vi "Orca Flash Capture Manager.vi"(7 "Calling VI Ref":refnum<vi>) -> ()   [LabVIEW 2016]
uses:
  Orca Flash Capture Manager Controls/Orca Flash Capture Switch Line Scan Modes.ctl
  Orca Flash Capture Manager Controls/Orca Flash Capture Line Scan Settings.ctl
  Orca Flash Capture Manager Controls/Orca Flash Switch Cycles Steps.ctl
  Orca Flash Capture Manager Controls/Orca Flash Channel Element.ctl
  <vilib>/Utility/miscctls.llb/LVPointTypeDef.ctl
  Orca Flash Capture Manager Controls/Orca Flash Capture Notifier Type.ctl
  Orca Flash Capture Manager Controls/Orca Flash Capture Actions.ctl
  <vilib>/vision/Image Controls.llb/IMAQ Image.ctl
  Orca Flash Capture Manager Controls/Orca Flash Capture Line Scan Filter Settings.ctl
  Device Library/Cameras/Hamamatsu/Orca Flash/Orca Flash Controls/Orca Flash SubRegion Type.ctl
  Hardware Configuration/Hardware Configuration Controls/Device Type.ctl
  Hardware Configuration/Hardware Configuration Controls/Device Function.ctl
  Device Library/Cameras/Hamamatsu/Orca Flash/Orca Flash Controls/Orca Flash Actions.ctl
  Device Library/Cameras/Hamamatsu/Orca Flash/Orca Flash Controls/Orca Flash Parameters.ctl
  Device Library/Cameras/Hamamatsu/Orca Flash/Orca Flash Controls/Orca Flash Parameter List.ctl
  Device Library/Cameras/Hamamatsu/Orca Flash/Orca Flash Controls/Orca Flash ROI.ctl
  Orca Flash Capture Manager Controls/Orca Flash Capture Cycle Step Count.ctl
  Device Manager/Common Device Queue/Common Device Controls/Common Device Actions.ctl
  Device Library/SMTP Email Alerts/SMTP Email Alerts Type Defs/SMTP Email Alerts Actions.ctl
  Device Library/DAQmx/AO Single Channel Triggered Ramp/AO SCTR Type Defs/AO SCTR Actions.ctl
  Wide Field Drift Correction/WFDC Controls/WFDC External Sync.ctl
  Wide Field Drift Correction/WFDC Controls/WFDC Cycle Pause.ctl
  Wide Field Drift Correction/WFDC Controls/WFDC Status.ctl
  Device Library/Stages/Stages Controls/Stage Actions.ctl
  Device Library/AOTF and AOM/AOTF Controls/AOTF Actions.ctl
  Device Library/Cameras/Camera Controls/Camera IMAQ Key Info.ctl
  <vilib>/Utility/file.llb/Read Delimited Spreadsheet (DBL).vi
  shell32.dll
panel:
  in  "Main Tab":T1(tab)
  in  "Scan Mode":T2=enum."Cycles Then Steps"
  out "Frame":u32(slide) scale=0.0..3.0
  out "Cycle":sgl(slide) scale=0.0..1.0
  in  "Base Save Path":path
  in  "Capture":bool
  in  "Live Preview":bool
  out "Z Step":sgl(slide) scale=0.0..1.0
  in  "File Name":string="Test Image"
  in  "Preview Exposure Time (s)":dbl=0.1 caption="Frame Rate (Hz)"
  in  "Capture Exposure Time (s)":dbl=0.1 caption="Frame Rate (Hz)"
  in  "No. of Frames":u32=1 min=1
  in  "No. of Cycles":u16=1 min=1
  in  "No. of Z Steps":u16=1 min=1
  in  "Z Step Size (µm)":dbl min=-10.0 max=10.0
  out "Current Cycle":u16
  out "Current Step":u16
  out "Current Frame":u32
  in  "Auto Update Subfolder":bool=TRUE
  in  "Subfolder Name":string="Area"
  in  "Channel Array":T3[](array[typedef])
  in  "Channels On/Off":bool
  in  "Current Filter":i32(ring) items=["Quad Band", "Cy3 / Cy5"]
  in  "Save As Preset":bool
  in  "Line Scan Active":bool
  in  "Number of Lines":u32=8 min=1 max=200 step=1
  in  "Line Scan Mode":T4
  in  "Line Scanning Presets":u16(ring) items=["04 FPS", "08 FPS Clean", "08 FPS", "40 FPS"]
  in  "Line Scan Settings":T5
  in  "Collect Metadata":bool
  in  "Edit Metadata":bool
  in  "Camera Settings":bool
  in  "Email Alerts":bool
  in  "Email Address":string
  in  "Auto Laser Off Time (min)":u16=30
  in  "Quit":bool
  # "Live Preview"
  # "Capture"
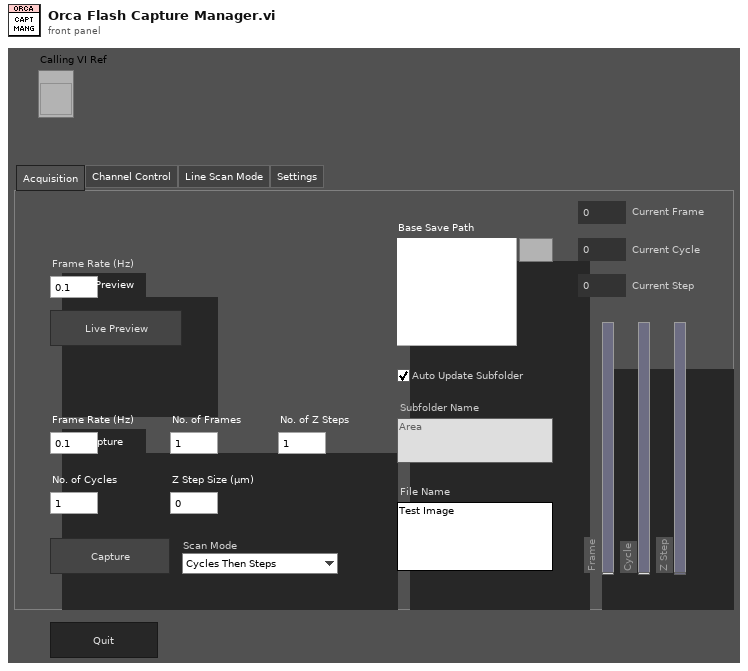
[diagram p1: front panel]
types:
  T1 = enum32{"Acquisition", "Channel Control", "Line Scan Mode", "Settings"}
  T2 = typedef "Orca Flash Switch Cycles Steps.ctl" = enum16{"Steps Then Cycles", "Cycles Then Steps"}
  T3 = typedef "Orca Flash Channel Element.ctl" = cluster{"On/Off":bool, "Name":string}
  T4 = typedef "Orca Flash Capture Switch Line Scan Modes.ctl" = enum32{"Automatic", "Use Presets", "Manual"}
  T5 = typedef "Orca Flash Capture Line Scan Settings.ctl" = cluster{"Interline Interval":dbl, "Offset (V)":dbl, "Amplitude (V)":dbl, "Samples Per Channel":dbl, "Delay (ms)":dbl}
  T6 = typedef "Orca Flash SubRegion Type.ctl" = cluster{"Name":string, "H Offset":i32, "V Offset":i32, "H Width":i32, "V Width":i32, "Active?":bool}
  T7 = typedef "IMAQ Image.ctl" = refnum<image>
  T8 = cluster{"Image Ref":T7, "Cycle Number":u16, "Camera Running?":bool, "Capture?":bool}
  T9 = typedef "Orca Flash Capture Line Scan Filter Settings.ctl" = cluster{"Filter Name":string, "Offset (V)":dbl}[]
  T10 = enum8{"Enabled", "Disabled", "Disabled and Grayed Out"}
  T11 = typedef "Orca Flash Capture Notifier Type.ctl" = cluster{"Actions":T12, "Running?":bool, "Preview Exposure (s)":dbl, "Capture Exposure (s)":dbl, "Cycles":u16, "Frames":u32, "No. of Z Steps":u16, "Z Step Size (µm)":dbl, "Base Path":path, "Init Z Position (µm)":dbl, "Save Path":path, "Line Scan?":bool, "Line Scan Mode":T4, "Collect Metadata?":bool}
  T12 = typedef "Orca Flash Capture Actions.ctl" = enum16{"Idle", "Live Preview", "Capture", "Laser On", "Laser Off", "Open Shutters", "Close Shutters", "Set Exposure Time", "Start Acquisition", "Update SubFolder", "Write Metadata", "Setup", "Camera", "Switch", "Step", "Cycle", "External Cycle Sync", "Abort", "Quit"}
  T13 = enum16{"Always On", "Always Off", "Off While Running"}
  T14 = typedef "LVPointTypeDef.ctl" = cluster{"Horizontal":i16, "Vertical":i16}
  T15 = typedef "Image Type" = u32
  T16 = typedef "Device Function.ctl" = enum16{"Primary", "Secondary", "Overview", "Wide Field Drift Correction", "642 nm Excitation", "560 nm Excitation", "546 nm Excitation", "488 nm Excitation", "405 nm Excitation", "Objective Drift Correction", "4Pi Objective Lock", "Objective XY", "Objective Z", "Sample XY", "Sample Coarse Z", "Sample Z", "4Pi Lower", "4Pi Upper", "Adj Cavity", "Line Scanning", "Alert"}
  T17 = typedef "Device Type.ctl" = enum16{"AOTF", "Camera", "Deformable Mirror", "Laser", "Shutter", "Stage", "Waveform", "Email"}
  T18 = typedef "Orca Flash ROI.ctl" = cluster{"H Offset":i32, "V Offset":i32, "H Width":i32, "V Width":i32}
  T19 = typedef "Orca Flash Parameters.ctl" = cluster{"Value":dbl, "Parameter":T20}
  T20 = typedef "Orca Flash Parameter List.ctl" = u32
  T21 = typedef "Orca Flash Actions.ctl" = enum16{"IDLE", "PREVIEW", "RECORD", "Record Settings", "SETPARAM", "GETPARAM", "SETROI", "GETROI", "PROGRESSIVE MODE", "AREA MODE", "STATUS", "QUIT"}
  T22 = typedef "Orca Flash Capture Cycle Step Count.ctl" = cluster{"Scan Mode":T2, "Current Step":u16, "Current Cycle":u16, "Num of Steps":u16, "Num of Cycles":u16}
  T23 = typedef "WFDC Status.ctl" = enum16{"Idle", "Busy", "DC Active", "Error"}
  T24 = typedef "WFDC External Sync.ctl" = cluster{"Cycle Sync":T25, "Z Offset":dbl, "WFDC Status":T23}
  T25 = typedef "WFDC Cycle Pause.ctl" = enum16{"Pause Requested", "Paused", "Resume Requested", "Resumed"}
  T26 = typedef "SMTP Email Alerts Actions.ctl" = enum16{"Set Recipient", "Send Message", "Quit"}
  T27 = typedef "Stage Actions.ctl" = enum16{"Get Position", "MVR", "MOVE", "HALT", "ONTARGET", "ERROR", "REFERENCE", "INIT", "VELOCITY", "STATUS", "EXIT", "HOME", "ZEROPOS", "NANOPOS", "ANALOG", "QUIT"}
  T28 = typedef "AOTF Actions.ctl" = enum16{"Error Check", "Blank", "Line On/Off", "Set Power", "Status", "Quit"}
  T29 = typedef "AO SCTR Actions.ctl" = enum16{"Stop at Offset", "Update and Run", "Quit"}
  T30 = typedef "Camera IMAQ Key Info.ctl" = cluster{"Frame":u32, "Sensor Height":i32, "Sensor Width":i32, "ROI Height":i32, "ROI Width":i32, "ROI Enable?":bool, "Bit per Pixel":u8}
  T31 = typedef "Common Device Actions.ctl" = enum16{"Specific Action", "Open Front Panel", "Close Front Panel", "Quit", "Quit All"}
  T32 = typedef "LVRectTypeDef.ctl" = cluster{"Left":i16, "Top":i16, "Right":i16, "Bottom":i16}
  T33 = typedef "LVBoundsTypeDef.ctl" = cluster{"Width":u32, "Height":u32}
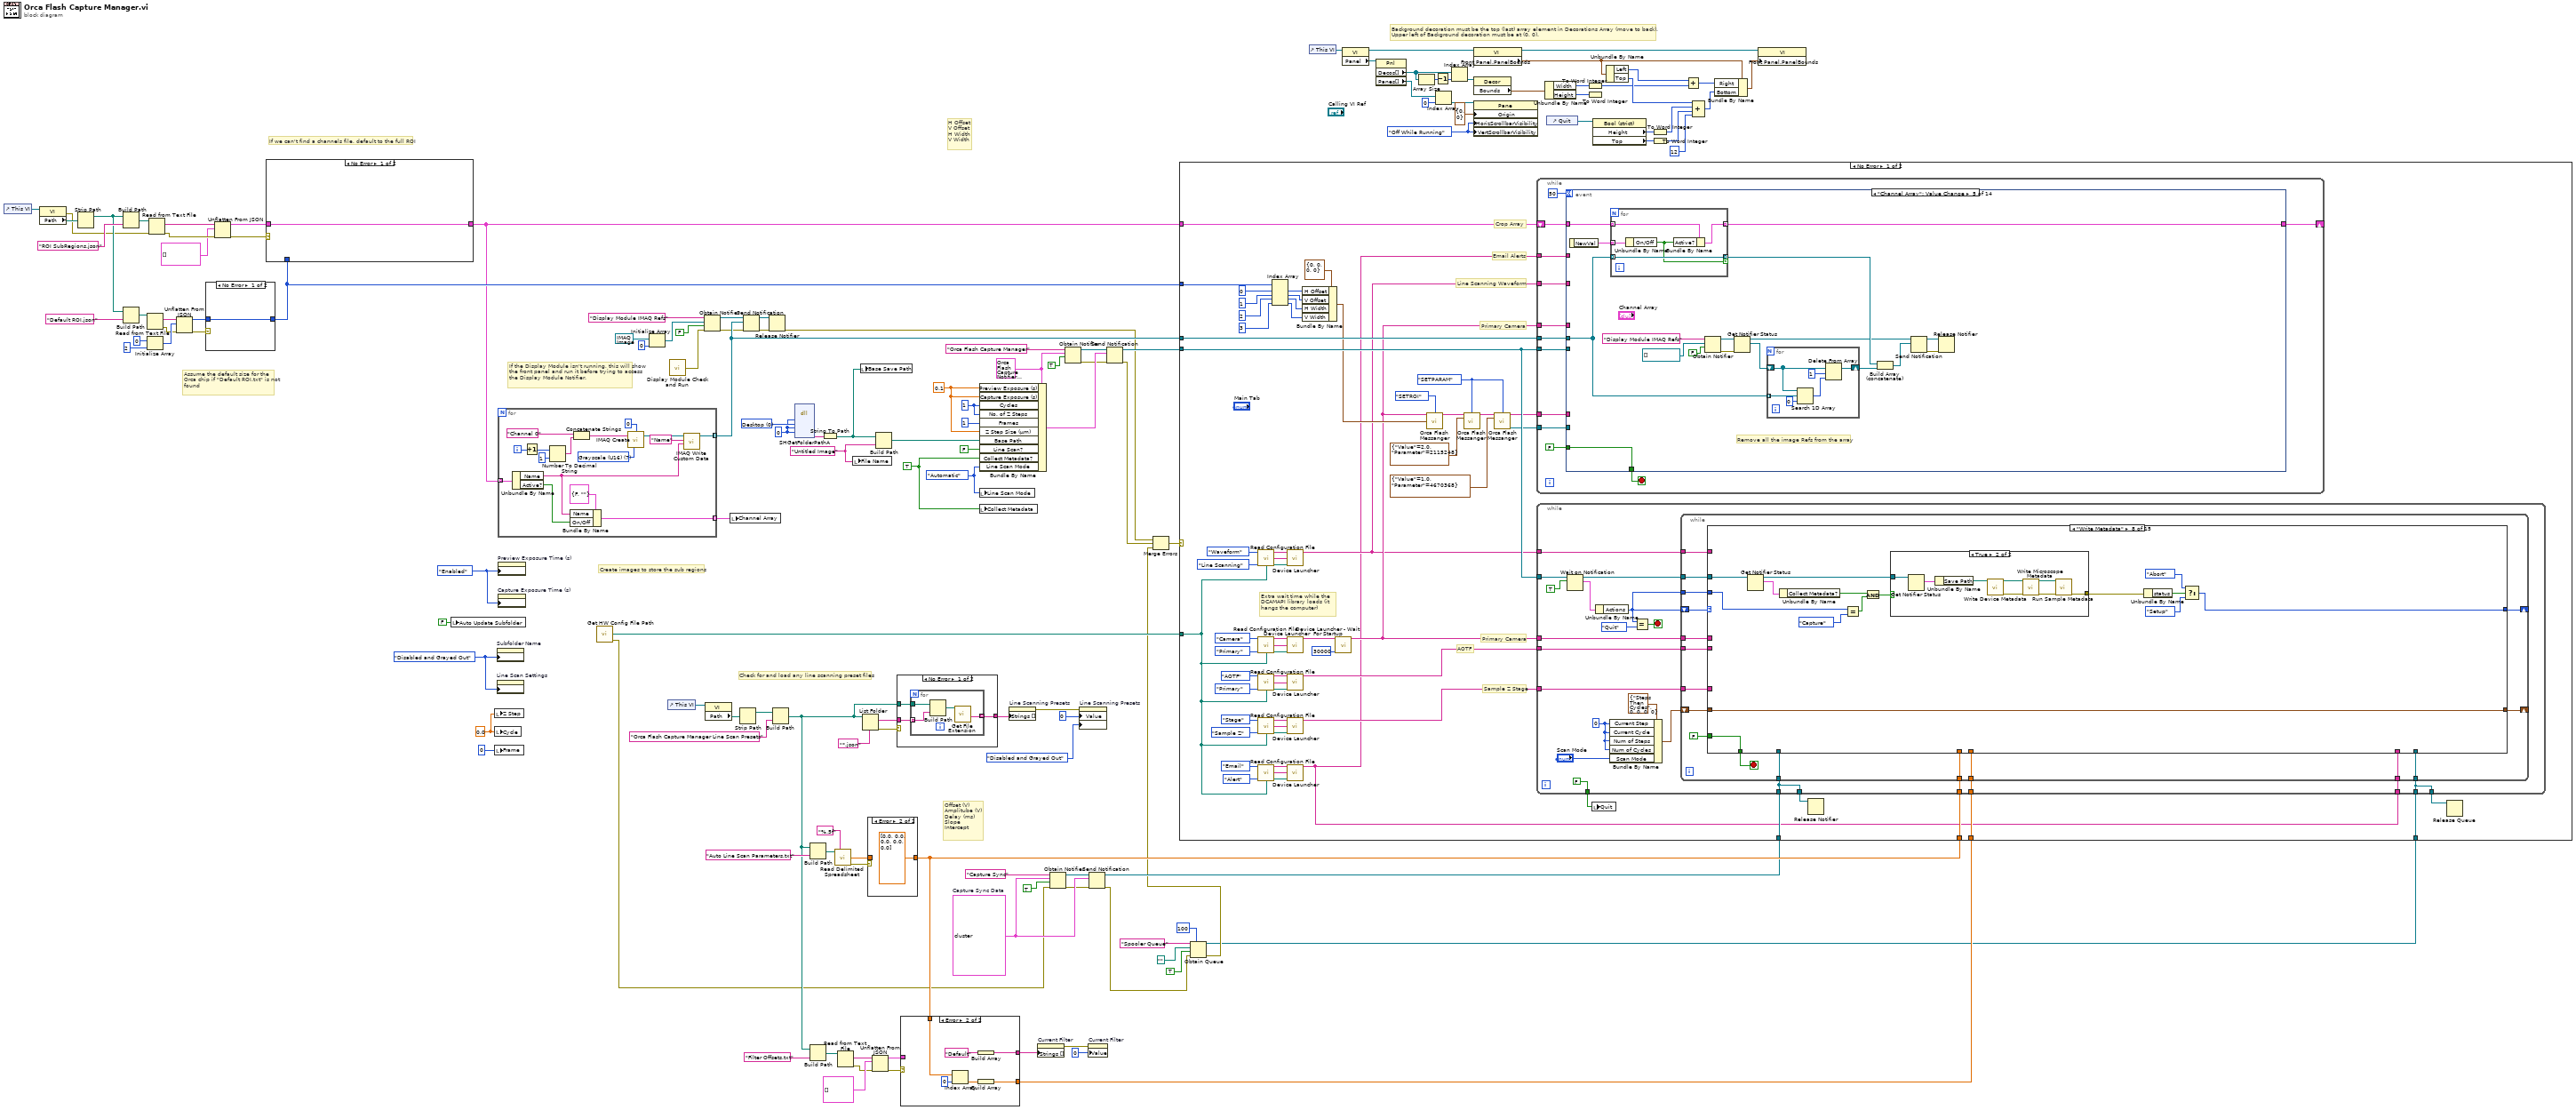
[diagram p0: block diagram]
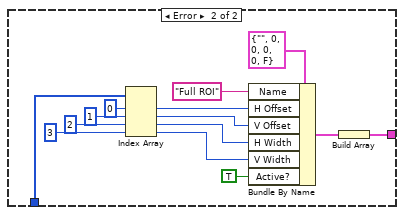
[diagram p2: hidden frame]
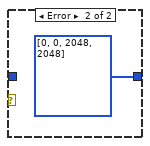
[diagram p3: hidden frame]
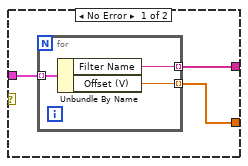
[diagram p4: hidden frame]
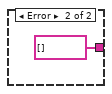
[diagram p6: hidden frame]
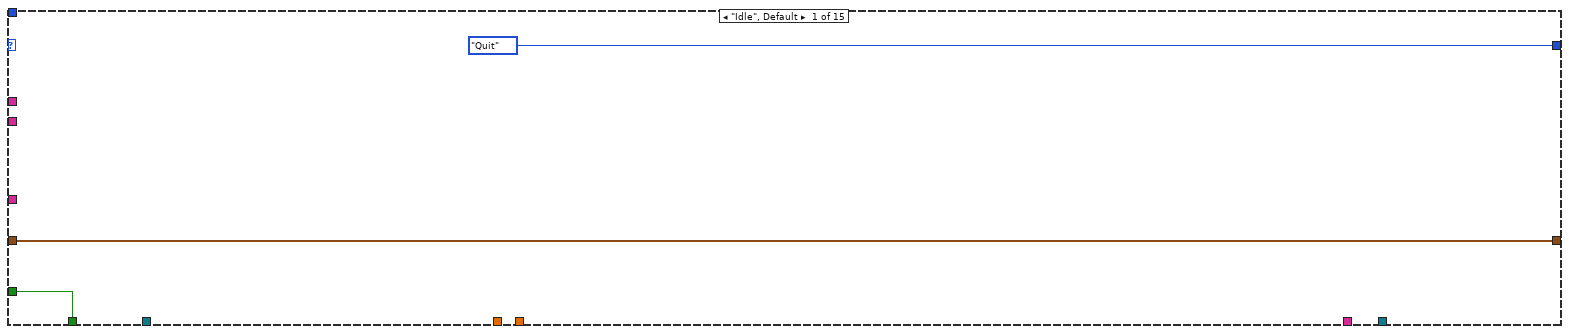
[diagram p7: hidden frame]
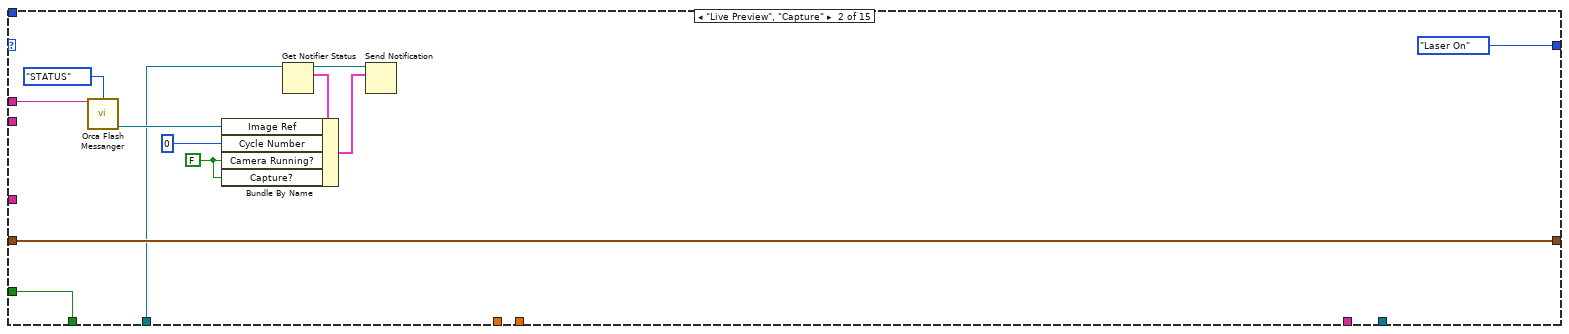
[diagram p8: hidden frame]
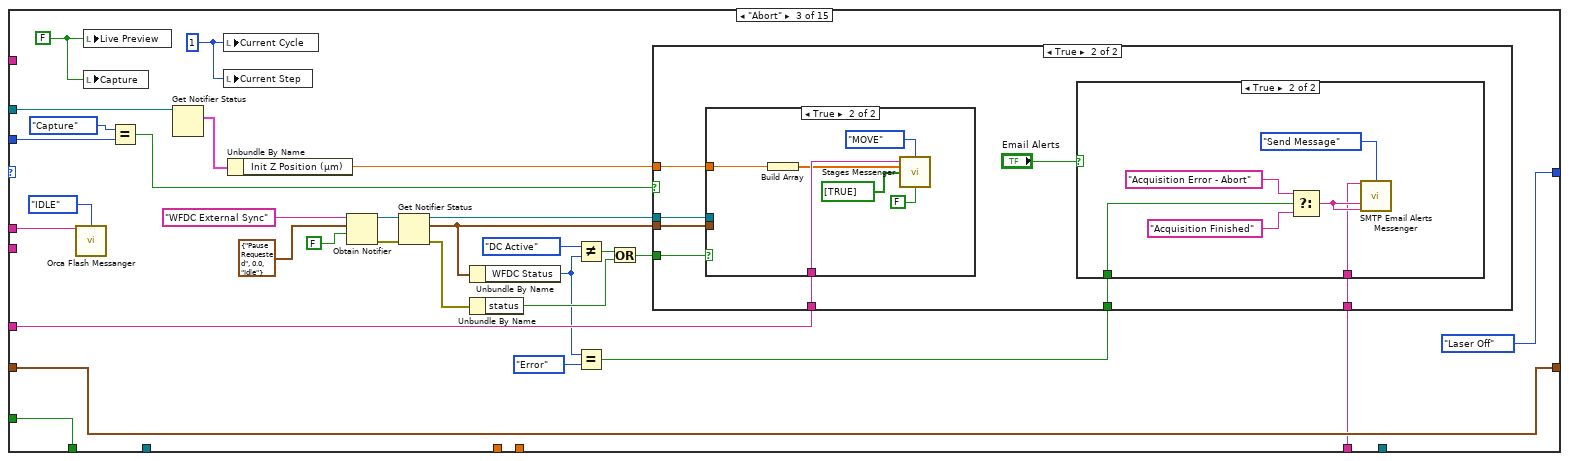
[diagram p9: hidden frame]
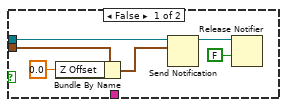
[diagram p12: hidden frame]
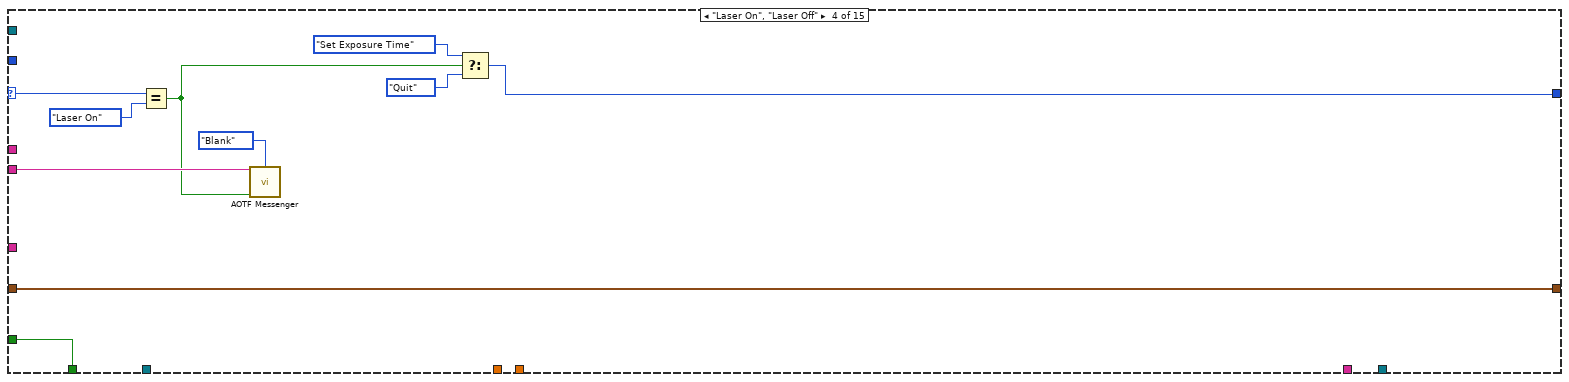
[diagram p13: hidden frame]
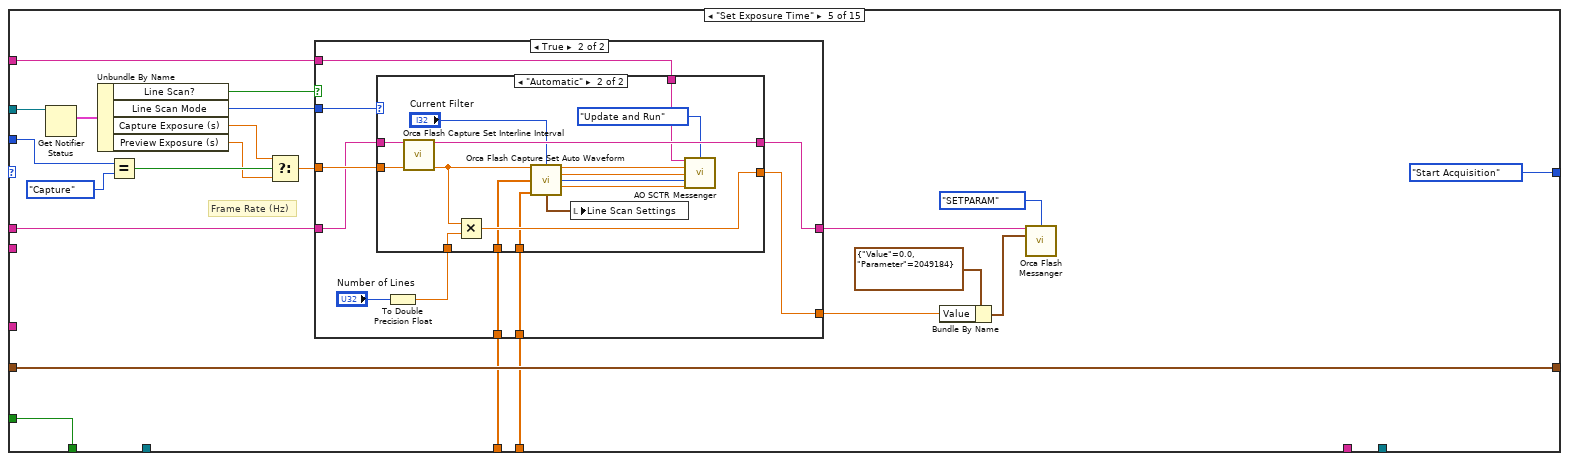
[diagram p14: hidden frame]
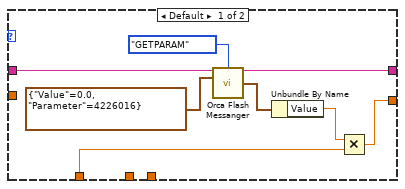
[diagram p16: hidden frame]
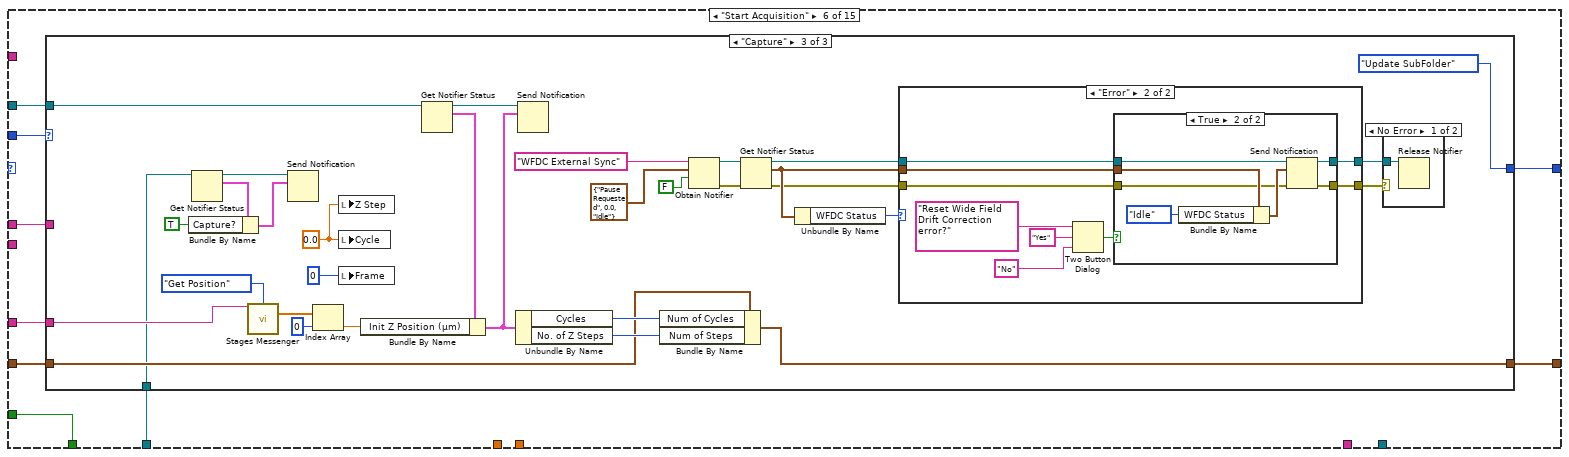
[diagram p17: hidden frame]
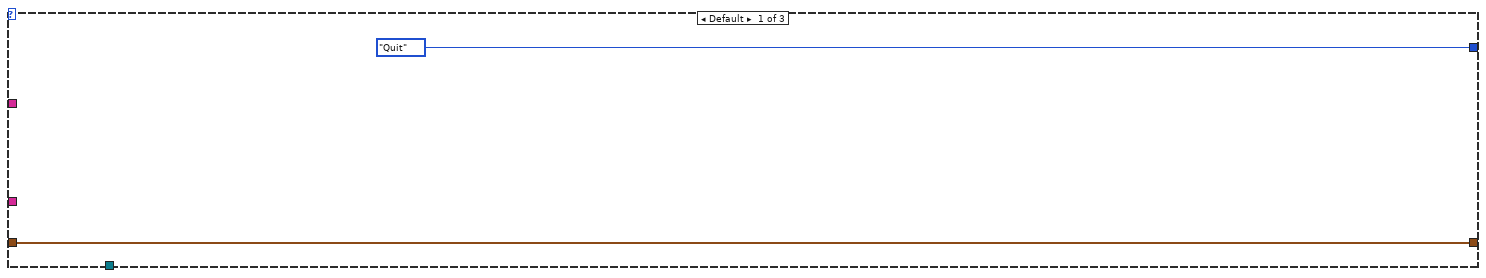
[diagram p18: hidden frame]
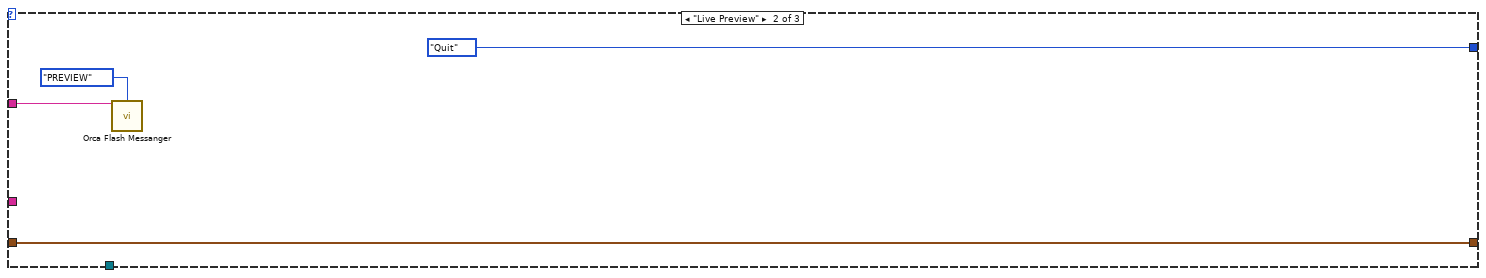
[diagram p19: hidden frame]
diagram:
  w16 = TRUE
  w22 = sgl 0.0 ("Cycle")
  w23 = T8 {"Image Ref"=refnum, "Cycle Number"=0, "Camera Running?"=FALSE, "Capture?"=FALSE}  # Capture Sync Data
  w45 = T10."Enabled" ("Disabled")
  w17 = Orca_Flash_Capture_Switch_Line_Scan_Modes."Automatic" ("Line Scan Mode")
  w46 = T10."Disabled and Grayed Out" ("Disabled")
  w87 = "Untitled Image"
  w90 = 0 items=["Desktop"=0, "Personal Documents"=5, "AppData"=26, "Local AppData"=28, "Common AppData"=35, "Program Files"=38, "Program Files Common"=43, "Common Documents"=46] ("Requested Path")
  w89 = 0 ("HWND")
  w94 = u16 1 ("Cycles")
  w92 = 0.1 ("Preview Exposure (s)")
  w96 = T11 {"Actions"=enum."Live Preview", "Running?"=FALSE, "Preview Exposure (s)"=0.1, "Capture Exposure (s)"=0.1, "Cycles"=1, "Frames"=0, "No. of Z Steps"=0, "Z Step Size (µm)"=0.0, "Base Path"=path "", "Init Z Position (µm)"=0.0, "Save Path"=path "", "Line Scan?"=FALSE, "Line Scan Mode"=enum."Automatic", "Collect Metadata?"=FALSE} ("4Pi Capture Notifier Type")
  w117 = T13."Off While Running" ("Vertical Scrollbar Visibility")
  # "If we can't find a channels file, default to the full ROI"
  # "Assume the default size for the Orca chip if \"Default ROI.txt\" is not found"
  # "Offset (V)\nAmplitube (V)\nDelay (ms)\nSlope\nIntercept"
  # "Check for and load any line scanning preset files"
  # "If the Display Module isn't running, this will show the front panel and run it before trying to access the Display Module Notifier."
  # "H Offset\nV Offset\nH Width\nV Width"
  # "Create images to store the sub regions"
  # "Background decoration must be the top (last) array element in Decorations Array (move to back).\nUpper left of Background decoration must be at (0, 0)."
  n1 = control-ref of="This VI"() -> (w99:refnum<vi>)
  n2 = property class="VI"(reference=w99) -> (error out=w72:errorcluster, "Path"=w98:path)  [unwired: 1 in, 1 out]
  n3 = Strip Path(path=w98) -> (stripped path=w82:path)  [unwired: 1 out]
  n4 = Build Path(base path=w82, name or relative path="ROI SubRegions.json") -> (appended path=w84:path)
  n5 = Build Path(base path=w82, name or relative path="Default ROI.json") -> (appended path=w80:path)
  n6 = Read from Text File(file (use dialog)=w80) -> (text=w79:string, error out=w73:errorcluster)  [unwired: 3 in, 2 out]
  n7 = Initialize Array(0 ("element"), 2 ("dimension size")) -> (w76:i32[])
  n8 = Read from Text File(file (use dialog)=w84, error in=w72) -> (text=w83:string, error out=w71:errorcluster)  [unwired: 2 in, 2 out]
  n9 = Unflatten From JSON(JSON string=w79, type and defaults=w76, error in (no error)=w73) -> (value=w6:i32[], error out=w7:errorcluster)  [unwired: 4 in]
  n10 = case shown="No Error" w7 {
    tunnel: w6 -> [w135 _]
    tunnel: [w135 i32[] [0, 0, 2048, 2048]] -> w3
    frame No Error {
    }
    frame Error {
    }
  }
  n11 = Unflatten From JSON(JSON string=w83, type and defaults=T6[] [], error in (no error)=w71) -> (value=w4:T6[], error out=w5:errorcluster)  [unwired: 4 in]
  n12 = case shown="No Error" w5 {
    tunnel: w4 -> [w137 _]
    tunnel: [w137 w148] -> w2
    tunnel: w3 -> [_ w147]
    frame No Error {
    }
    frame Error {
      n13 = Index Array(array=w147, index #1=0 ("index"), index #2=1 ("index"), index #3=2 ("index"), index #4=3 ("index")) -> (element #1=w142:i32, element #2=w141:i32, element #3=w140:i32, element #4=w139:i32)
      n14 = Bundle By Name(cluster=T6 {"Name"="", "H Offset"=0, "V Offset"=0, "H Width"=0, "V Width"=0, "Active?"=FALSE} ("ROI Sub Region"), "Name"="Full ROI", "H Offset"=w142, "V Offset"=w141, "H Width"=w140, "V Width"=w139, "Active?"=TRUE) -> (w149:T6)
      n15 = Build Array(w149) -> (w148:T6[])
    }
  }
  n16 = local write "Auto Update Subfolder"(FALSE ("Auto Update Subfolder")) -> ()
  n17 = local write "Z Step"(w22) -> ()
  n18 = local write "Cycle"(w22) -> ()
  n19 = local write "Frame"(u32 0 ("Frame")) -> ()
  n20 = property on="Subfolder Name" class="Str"("DisabledEnum"=w46) -> ()  [unwired: 2 in, 2 out]
  n21 = property on="Line Scan Settings" class="Clust (strict)"("DisabledEnum"=w46) -> ()  [unwired: 2 in, 2 out]
  n22 = property on="Preview Exposure Time (s)" class="DigNum (strict)"("DisabledEnum"=w45) -> ()  [unwired: 2 in, 2 out]
  n23 = property on="Capture Exposure Time (s)" class="DigNum (strict)"("DisabledEnum"=w45) -> ()  [unwired: 2 in, 2 out]
  n24 = for {
    tunnel: [w157] -> w100 mode=indexing
    tunnel: w2 -> [w159] mode=indexing
    tunnel: [w153] -> w1 mode=indexing
    i -> [w167]
    w162 = T15 7 items=["Grayscale (U8)", "Grayscale (I16)", "Grayscale (SGL)", "Complex (CSG)", "RGB (U32)", "HSL (U32)", "RGB (U64)", "Grayscale (U16)"] ("Image Type")
    n25 = Unbundle By Name(w159) -> ("Name"=w154:string, "Active?"=w152:bool)
    n26 = Increment(x=w167) -> (x+1=w165:i32)
    n27 = Number To Decimal String(number=w165, width (-)=i16 1) -> (decimal integer string=w163:string)
    n28 = Bundle By Name(cluster=T3 {"On/Off"=FALSE, "Name"=""} ("Channel Control Cluster"), "Name"=w154, "On/Off"=w152) -> (w153:T3)
    n29 = Concatenate Strings("Channel 0" ("name (unnamed)"), w163) -> (w160:string)
    n30 = call "IMAQ Create"("Border Size"=0, "Image Name"=w160, "Image Type"=w162) -> ("New Image"=w158:T7)  [unwired: 2 in, 1 out]
    n31 = call "IMAQ Write Custom Data"("Custom Data In"=w154, "Key"="Name", "Image"=w158) -> ("Image Out"=w157:T7)  [unwired: 7 in, 1 out]
  }
  n32 = call "Get HW Config File Path.vi"() -> ("File Path"=w60:path, "Error"=w20:errorcluster)  [unwired: 14 in]
  n33 = Initialize Array(T7 refnum ("New Image"), 0 ("dimension size")) -> (w62:T7[])
  n34 = control-ref of="This VI"() -> (w57:refnum<vi>)
  n35 = call "Display Module Check and Run.vi"() -> ("Error"=w61:errorcluster)  [unwired: 15 in]
  n36 = Obtain Notifier(name (unnamed)="Display Module IMAQ Refs", notification data type=w62, create if not found? (T)=FALSE, error in (no error)=w61) -> (notifier out=w101:refnum<notifier>, error out=w70:errorcluster)  [unwired: 1 out]
  n37 = property class="VI"(reference=w57) -> ("Path"=w56:path)  [unwired: 1 in, 2 out]
  n38 = local write "Channel Array"(w1) -> ()
  n39 = Strip Path(path=w56) -> (stripped path=w55:path)  [unwired: 1 out]
  n40 = Send Notification(notification=w100, notifier=w101, error in (no error)=w70) -> (notifier out=w85:refnum<notifier>, error out=w75:errorcluster)
  n41 = Release Notifier(notifier=w85, error in (no error)=w75) -> (error out=w67:errorcluster)  [unwired: 1 in, 2 out]
  n42 = Build Path(base path=w55, name or relative path="Orca Flash Capture Manager Line Scan Presets") -> (appended path=w39:path)
  n43 = dll-call lib="shell32.dll" fn="SHGetFolderPathA"("HWND"=w89, "nFolder"=w90, "hToken"=w89, "dwFlags"=w89) -> ("pszPath"=w88:string)  [unwired: 9 in, 2 out]
  n44 = Build Path(base path=w39, name or relative path="Auto Line Scan Parameters.txt") -> (appended path=w43:path)
  n45 = Build Path(base path=w39, name or relative path="Filter Offsets.txt") -> (appended path=w37:path)
  n46 = String To Path(string=w88) -> (path=w86:path)
  n47 = call-poly <vilib>:"Read Delimited Spreadsheet.vi"("file path (dialog if empty)"=w43, "format (%.3f)"="%.5f") -> ("first row"=w40:dbl[], "error out"=w41:errorcluster)  [unwired: 8 in, 4 out]
  n48 = Read from Text File(file (use dialog)=w37) -> (text=w36:string, error out=w34:errorcluster)  [unwired: 3 in, 2 out]
  n49 = local write "File Name"(w87) -> ()
  n50 = local write "Base Save Path"(w86) -> ()
  n51 = List Folder(path=w39, pattern="*.json") -> (filenames=w52:string[], error out=w51:errorcluster)  [unwired: 2 in, 2 out]
  n52 = case shown="Error" w41 {
    tunnel: w40 -> [w168 _]
    tunnel: [w168 dbl[] [0.0, 0.0, 0.0, 0.0, 0.0] ("first row")] -> w31
    frame No Error {
    }
    frame Error {
    }
  }
  n53 = Unflatten From JSON(JSON string=w36, type and defaults=T9 [] ("Line Scan Filter Parameters"), error in (no error)=w34) -> (value=w33:T9, error out=w32:errorcluster)  [unwired: 4 in]
  n54 = Build Path(base path=w86, name or relative path=w87) -> (appended path=w91:path)
  n55 = case shown="No Error" w51 {
    tunnel: w52 -> [w172 _]
    tunnel: w39 -> [w171 _]
    tunnel: [w170 string[] []] -> w50
    frame No Error {
      n56 = for {
        tunnel: w172 -> [w175] mode=indexing
        tunnel: w171 -> [w176]
        tunnel: [w173] -> w170 mode=indexing
        n57 = Build Path(base path=w176, name or relative path=w175) -> (appended path=w174:path)
        n58 = call <vilib>:"Get File Extension.vi"("file"=w174) -> ("filename without extension"=w173:string)  [unwired: 6 in, 4 out]
      }
    }
    frame Error {
    }
  }
  n59 = case shown="Error" w32 {
    tunnel: w33 -> [w180 _]
    tunnel: w31 -> [_ w188]
    tunnel: [w179 w185] -> w30
    tunnel: [w178 w184] -> w27
    frame No Error {
      n60 = for {
        tunnel: w180 -> [w183] mode=indexing
        tunnel: [w182] -> w179 mode=indexing
        tunnel: [w181] -> w178 mode=indexing
        n61 = Unbundle By Name(w183) -> ("Filter Name"=w182:string, "Offset (V)"=w181:dbl)
      }
    }
    frame Error {
      n62 = Index Array(array=w188, index=0) -> (element=w186:dbl)
      n63 = Build Array("Default") -> (w185:string[])
      n64 = Build Array(w186) -> (w184:dbl[])
    }
  }
  n65 = Bundle By Name(cluster=w96, "Preview Exposure (s)"=w92, "Capture Exposure (s)"=w92, "Cycles"=w94, "No. of Z Steps"=w94, "Frames"=u32 1, "Z Step Size (µm)"=w92, "Base Path"=w91, "Line Scan?"=FALSE, "Collect Metadata?"=w16, "Line Scan Mode"=w17) -> (w95:T11)
  n66 = local write "Line Scan Mode"(w17) -> ()
  n67 = local write "Collect Metadata"(w16) -> ()
  n68 = property on="Line Scanning Presets" class="Ring (strict)"("Strings []"=w50) -> (error out=w49:errorcluster)  [unwired: 2 in, 1 out]
  n69 = property on="Current Filter" class="Ring (strict)"("Strings []"=w30) -> (error out=w29:errorcluster)  [unwired: 2 in, 1 out]
  n70 = Obtain Notifier(name (unnamed)="Capture Sync", notification data type=w23, create if not found? (T)=TRUE, error in (no error)=w20) -> (notifier out=w24:refnum<notifier>, error out=w19:errorcluster)  [unwired: 1 out]
  n71 = Obtain Notifier(name (unnamed)="Orca Flash Capture Manager", notification data type=w96, create if not found? (T)=TRUE) -> (notifier out=w103:refnum<notifier>, error out=w74:errorcluster)  [unwired: 1 in, 1 out]
  n72 = property on="Line Scanning Presets" class="Ring (strict)"(error in=w49, "Value"=u16 0, "DisabledEnum"=T10."Disabled and Grayed Out" ("Disabled")) -> ()  [unwired: 1 in, 2 out]
  n73 = property on="Current Filter" class="Ring (strict)"(error in=w29, "Value"=0) -> ()  [unwired: 1 in, 2 out]
  n74 = Send Notification(notification=w23, notifier=w24, error in (no error)=w19) -> (notifier out=w18:refnum<notifier>, error out=w11:errorcluster)
  n75 = Send Notification(notification=w95, notifier=w103, error in (no error)=w74) -> (notifier out=w102:refnum<notifier>, error out=w68:errorcluster)
  n76 = Obtain Queue(max queue size (-1, unlimited)=100, name (unnamed)="Spooler Queue", element data type=path "", create if not found? (T)=TRUE, error in (no error)=w11) -> (queue out=w9:refnum<queue>, error out=w10:errorcluster)  [unwired: 1 out]
  n77 = Merge Errors(w67, w68, w10) -> (w69:errorcluster)
  n78 = case shown="No Error" w69 {
    tunnel: w60 -> [w193 _]
    tunnel: w102 -> [w241 w1194]
    tunnel: w100 -> [w231 w1192]
    tunnel: w2 -> [w230 _]
    tunnel: w3 -> [w221 _]
    tunnel: w31 -> [w202 _]
    tunnel: w27 -> [w201 _]
    tunnel: w18 -> [w200 _]
    tunnel: w9 -> [w191 _]
    frame No Error {
      w226 = Orca_Flash_Actions."SETPARAM" ("Camera Actions")
      # "Crop Array"
      # "Email Alerts"
      # "Line Scanning Waveform"
      # "Primary Camera"
      # "Extra wait time while the DCAMAPI library loads (it hangs the computer)"
      # "Sample Z Stage"
      # "AOTF"
      # "Primary Camera"
      n79 = call "Read Configuration File.vi"("Device Type"=Device_Type."Waveform", "Device Function"=Device_Function."Line Scanning", "Config File Path"=w193) -> ("Unique Notifier Name"=w206:string, "Device Ports/IDs/Channels"=w207:string[], "Device Engine Path"=w204:path)  [unwired: 9 in, 1 out]
      n80 = call "Read Configuration File.vi"("Device Type"=Device_Type."Camera", "Device Function"=Device_Function."Primary", "Config File Path"=w193) -> ("Unique Notifier Name"=w251:string, "Device Ports/IDs/Channels"=w250:string[], "Device Engine Path"=w249:path)  [unwired: 9 in, 1 out]
      n81 = call "Read Configuration File.vi"("Device Type"=Device_Type."AOTF", "Device Function"=Device_Function."Primary", "Config File Path"=w193) -> ("Unique Notifier Name"=w242:string, "Device Ports/IDs/Channels"=w243:string[], "Device Engine Path"=w244:path)  [unwired: 9 in, 1 out]
      n82 = call "Read Configuration File.vi"("Device Type"=Device_Type."Stage", "Device Function"=Device_Function."Sample Z", "Config File Path"=w193) -> ("Unique Notifier Name"=w238:string, "Device Ports/IDs/Channels"=w236:string[], "Device Engine Path"=w235:path)  [unwired: 9 in, 1 out]
      n83 = call "Read Configuration File.vi"("Device Type"=Device_Type."Email", "Device Function"=Device_Function."Alert", "Config File Path"=w193) -> ("Unique Notifier Name"=w196:string, "Device Ports/IDs/Channels"=w195:string[], "Device Engine Path"=w198:path)  [unwired: 9 in, 1 out]
      n84 = Index Array(array=w221, index #1=0 ("index"), index #2=1 ("index"), index #3=2 ("index"), index #4=3 ("index")) -> (element #1=w216:i32, element #2=w213:i32, element #3=w214:i32, element #4=w215:i32)
      n85 = call "Device Launcher.vi"("Notifier Name"=w206, "Device Ports/IDs/Channels"=w207, "Device Engine Path"=w204) -> ("Notifier Name"=w203:string)  [unwired: 11 in, 1 out]
      n86 = call "Device Launcher.vi"("Notifier Name"=w251, "Device Ports/IDs/Channels"=w250, "Device Engine Path"=w249) -> ("Notifier Name"=w210:string)  [unwired: 11 in, 1 out]
      n87 = call "Device Launcher.vi"("Notifier Name"=w242, "Device Ports/IDs/Channels"=w243, "Device Engine Path"=w244) -> ("Notifier Name"=w240:string)  [unwired: 11 in, 1 out]
      n88 = call "Device Launcher.vi"("Notifier Name"=w238, "Device Ports/IDs/Channels"=w236, "Device Engine Path"=w235) -> ("Notifier Name"=w233:string)  [unwired: 11 in, 1 out]
      n89 = call "Device Launcher.vi"("Notifier Name"=w196, "Device Ports/IDs/Channels"=w195, "Device Engine Path"=w198) -> ("Notifier Name"=w192:string)  [unwired: 11 in, 1 out]
      n90 = Bundle By Name(cluster=T18 {"H Offset"=0, "V Offset"=0, "H Width"=0, "V Width"=0} ("Orca Flash ROI"), "H Offset"=w216, "V Offset"=w213, "H Width"=w214, "V Width"=w215) -> (w212:T18)
      n91 = call "Device Launcher - Wait For Startup.vi"("Notifier Name"=w210, "Wait Time (ms)"=30000) -> ("Notifier Name (Dup)"=w209:string)  [unwired: 12 in, 1 out]
      n92 = call "Orca Flash Messanger.vi"("Notifier Name"=w209, "Camera Actions"=Orca_Flash_Actions."SETROI", "sCMOS ROI"=w212) -> ("Notifier Name Dup"=w229:string)  [unwired: 8 in, 4 out]
      n93 = call "Orca Flash Messanger.vi"("Notifier Name"=w229, "Camera Actions"=w226, "sCMOS Parameter"=T19 {"Value"=2.0, "Parameter"=2115248}) -> ("Notifier Name Dup"=w228:string)  [unwired: 8 in, 4 out]
      n94 = call "Orca Flash Messanger.vi"("Notifier Name"=w228, "Camera Actions"=w226, "sCMOS Parameter"=T19 {"Value"=1.0, "Parameter"=4670368}) -> ("Notifier Name Dup"=w227:string, "Image Ref"=w223:T7)  [unwired: 8 in, 3 out]
      n95 = while {
        tunnel: w241 -> [w801]
        tunnel: w227 -> [w800]
        tunnel: w223 -> [w798]
        tunnel: w231 -> [w797]
        shift-right: [w795] -> _
        shift-left: w230 -> [w796]
        tunnel: w209 -> [w794]
        tunnel: w203 -> [w793]
        tunnel: w192 -> [w792]
        stop <- w803 stop-if-true
        n96 = event shown="[4] \"Channel Array\": Value Change" {
          selector: _ -> [_ _ _ _ _ _ _ _ _ _ _ _ _ _]
          dyn-events: _ -> [_ _ _ _ _ _ _ _ _ _ _ _ _ _]
          timeout: 50 -> [_ _ _ _ _ _ _ _ _ _ _ _ _ _]
          tunnel: [w824 w856 w932 w954 w1021 w1038 w1063 w1085 w1101 w1125 w1149 w1166 w1175 w1190] -> w803
          tunnel: FALSE -> [w824 w856 w932 w954 w1021 w1038 w1063 w1085 w1101 w1125 w1149 w1166 w1175 _]
          tunnel: w801 -> [w820 w853 w929 _ _ _ w1057 w1083 _ w1123 _ _ w1170 w1189]
          tunnel: w800 -> [_ w852 _ _ _ _ _ _ _ _ _ _ _ _]
          tunnel: w798 -> [w822 _ _ w938 _ _ _ _ _ _ _ _ _ _]
          tunnel: w797 -> [w823 _ _ w944 w1014 _ _ _ _ _ _ _ _ w1177]
          tunnel: w796 -> [w804 w851 w921 w937 w1012 w1033 w1040 w1084 w1102 w1124 w1141 w1167 w1174 w1176]
          tunnel: [w804 w851 w921 w936 w1011 w1033 w1040 w1084 w1102 w1124 w1141 w1167 w1174 w1176] -> w795
          tunnel: w794 -> [_ _ _ _ _ _ w1051 _ _ w1109 _ _ _ _]
          tunnel: w793 -> [_ _ _ _ _ _ w1041 _ _ w1117 _ _ _ _]
          tunnel: w792 -> [_ w850 _ _ _ _ _ _ _ _ _ _ _ _]
          event Timeout {
            # "Turn all laser emission off if capture ends and no activity for X minutes."
            # "Convert to array and then crop. If you\nextract or mask image the destination\nimage custom data keys are overwritten."
            n97 = event-data() -> ()  [unwired: 1 in, 1 out]
            n98 = call "IMAQ ImageToArray"("Image"=w822) -> ("Image Pixels (U16)"=w821:u16[][])  [unwired: 3 in, 4 out]
            n99 = for {
              tunnel: w823 -> [w841] mode=indexing
              tunnel: w821 -> [w842]
              tunnel: w804 -> [w840] mode=indexing
              n100 = Unbundle By Name(w840) -> ("H Offset"=w839:i32, "H Width"=w838:i32, "V Offset"=w837:i32, "V Width"=w836:i32, "Active?"=w835:bool)
              n101 = case shown="True" w835 {
                tunnel: w842 -> [_ w849]
                tunnel: w841 -> [_ w848]
                tunnel: w839 -> [_ w846]
                tunnel: w838 -> [_ w845]
                tunnel: w837 -> [_ w844]
                tunnel: w836 -> [_ w843]
                frame False {
                }
                frame True {
                  n102 = Array Subset(array=w849, index (row)=w846, length (row)=w845, index (col)=w844, length (col)=w843) -> (w847:u16[][])
                  n103 = call "IMAQ ArrayToImage"("Image Pixels (U16)"=w847, "Image"=w848) -> ()  [unwired: 8 in, 2 out]
                }
              }
            }
            n104 = Get Notifier Status(notifier=w820) -> (current notification=w819:T11, # waiting=w818:i32)  [unwired: 1 in, 3 out]
            n105 = Greater Than 0?(x=w818) -> (x > 0?=w817:bool)
            n106 = Unbundle By Name(w819) -> ("Running?"=w808:bool)
            n107 = feedback-in #1(w808) -> ()
            n108 = feedback #1(FALSE) -> (w815:bool)
            n109 = Not(x=w808) -> (.not. x?=w806:bool)
            n110 = Less?(x=w808, y=w815) -> (x < y?=w814:bool)
            n111 = And(x=w814, y=w817) -> (x .and. y?=w811:bool)
            n112 = feedback #2(FALSE) -> (w809:bool)
            n113 = case shown="True" w809 {
              tunnel: [FALSE w829] -> w805
              frame False {
              }
              frame True {
                n114 = feedback #3(u16 0) -> (w833:u16)
                n115 = Multiply(x="Auto Laser Off Time (min)", y=u16 1200) -> (x*y=w826:u16)
                n116 = Increment(x=w833) -> (x+1=w830:u16)
                n117 = Equal?(x=w826, y=w830) -> (x = y?=w829:bool)
                n118 = Select(t=u16 0, s=w829, f=w830) -> (s? t:f=w831:u16)
                n119 = feedback-in #3(w831) -> ()
              }
            }
            n120 = Exclusive Or(1:w805, 2:w811) -> (0:w812:bool)
            n121 = Select(t=w811, s=w812, f=w809) -> (s? t:f=w810:bool)
            n122 = feedback-in #2(w810) -> ()
            n123 = And(x=w805, y=w806) -> (x .and. y?=w807:bool)
            n124 = case shown="True" w807 {
              frame False {
              }
              frame True {
                n125 = call "All Laser Emission Off.vi"() -> ()  [unwired: 16 in]
              }
            }
          }
          event "Camera Settings", "Preview Exposure Time (s)", "Capture Exposure Time (s)", "No. of Cycles", "No. of Frames", "No. of Z Steps", "Z Step Size (µm)", "Base Save Path", "File Name", "Email Address": Value Change {
            n126 = event-data() -> ("CtlRef"=w855:refnum<vi>)  [unwired: 1 in]
            n127 = property class="Ctl"(reference=w855) -> ("Label.Text"=w854:string)  [unwired: 1 in, 2 out]
            n128 = case shown="\"Base Save Path\", \"File Name\"" w854 {
              tunnel: w853 -> [_ w860 w868 w874 w880 w892 _ w908 w917 _]
              tunnel: w852 -> [_ _ _ _ _ _ w900 _ _ _]
              tunnel: w850 -> [_ _ _ _ _ _ _ _ _ w918]
              frame Default {
              }
              frame "No. of Cycles" {
                n129 = Get Notifier Status(notifier=w860) -> (notifier out=w859:refnum<notifier>, current notification=w861:T11)  [unwired: 1 in, 3 out]
                n130 = Bundle By Name(cluster=w861, "Cycles"="No. of Cycles", "Actions"=Orca_Flash_Capture_Actions."Idle") -> (w862:T11)
                n131 = Send Notification(notification=w862, notifier=w859) -> ()  [unwired: 1 in, 2 out]
              }
              frame "No. of Frames" {
                n132 = To Double Precision Float(number="No. of Frames") -> (double precision float=w864:dbl)
                n133 = property on="Frame" class="Slide (strict)"("Scale.Maximum"=w864, "Scale.Minimum"=0.0 ("Scale.Range:Minimum")) -> ()  [unwired: 2 in, 2 out]
                n134 = Get Notifier Status(notifier=w868) -> (notifier out=w867:refnum<notifier>, current notification=w869:T11)  [unwired: 1 in, 3 out]
                n135 = Bundle By Name(cluster=w869, "Frames"="No. of Frames", "Actions"=Orca_Flash_Capture_Actions."Idle") -> (w870:T11)
                n136 = Send Notification(notification=w870, notifier=w867) -> ()  [unwired: 1 in, 2 out]
              }
              frame "No. of Z Steps" {
                n137 = Get Notifier Status(notifier=w874) -> (notifier out=w873:refnum<notifier>, current notification=w875:T11)  [unwired: 1 in, 3 out]
                n138 = Bundle By Name(cluster=w875, "No. of Z Steps"="No. of Z Steps", "Actions"=Orca_Flash_Capture_Actions."Idle") -> (w876:T11)
                n139 = Send Notification(notification=w876, notifier=w873) -> ()  [unwired: 1 in, 2 out]
              }
              frame "Z Step Size (µm)" {
                n140 = Get Notifier Status(notifier=w880) -> (notifier out=w879:refnum<notifier>, current notification=w881:T11)  [unwired: 1 in, 3 out]
                n141 = Bundle By Name(cluster=w881, "Z Step Size (µm)"="Z Step Size (µm)", "Actions"=Orca_Flash_Capture_Actions."Idle") -> (w882:T11)
                n142 = Send Notification(notification=w882, notifier=w879) -> ()  [unwired: 1 in, 2 out]
              }
              frame "Base Save Path", "File Name" {
                n143 = Path To String(path="Base Save Path") -> (string=w887:string)
                n144 = Equal?(x="", y=w887) -> (x = y?=w885:bool)
                n145 = case shown="True" w885 {
                  tunnel: [w895 w896] -> w884
                  tunnel: "Base Save Path" -> [w895 _]
                  frame False {
                  }
                  frame True {
                    w899 = 0 items=["Desktop"=0, "Personal Documents"=5, "AppData"=26, "Local AppData"=28, "Common AppData"=35, "Program Files"=38, "Program Files Common"=43, "Common Documents"=46] ("Requested Path")
                    w898 = 0 ("HWND")
                    n146 = dll-call lib="shell32.dll" fn="SHGetFolderPathA"("HWND"=w898, "nFolder"=w899, "hToken"=w898, "dwFlags"=w898) -> ("pszPath"=w897:string)  [unwired: 9 in, 2 out]
                    n147 = String To Path(string=w897) -> (path=w896:path)
                  }
                }
                n148 = Build Path(base path=w884, name or relative path="File Name") -> (appended path=w888:path)
                n149 = Get Notifier Status(notifier=w892) -> (notifier out=w891:refnum<notifier>, current notification=w893:T11)  [unwired: 1 in, 3 out]
                n150 = Bundle By Name(cluster=w893, "Base Path"=w888, "Actions"=Orca_Flash_Capture_Actions."Idle") -> (w894:T11)
                n151 = Send Notification(notification=w894, notifier=w891) -> ()  [unwired: 1 in, 2 out]
              }
              frame "Camera Settings" {
                n152 = Select(t=Common_Device_Actions."Open Front Panel" ("Common Actions"), s="Camera Settings", f=Common_Device_Actions."Close Front Panel" ("Common Actions")) -> (s? t:f=w904:T31)
                n153 = call "Common Device Queue Messenger.vi"("Common Action"=w904, "Notifier Name"=w900) -> ()  [unwired: 13 in, 1 out]
              }
              frame "Preview Exposure Time (s)" {
                # "Add in a preview stop\nand restart here"
                n154 = Get Notifier Status(notifier=w908) -> (notifier out=w911:refnum<notifier>, current notification=w910:T11)  [unwired: 1 in, 3 out]
                n155 = Bundle By Name(cluster=w910, "Preview Exposure (s)"="Preview Exposure Time (s)", "Running?"=FALSE ("Abort"), "Actions"=Orca_Flash_Capture_Actions."Idle") -> (w909:T11)
                n156 = Send Notification(notification=w909, notifier=w911) -> ()  [unwired: 1 in, 2 out]
              }
              frame "Capture Exposure Time (s)" {
                n157 = Get Notifier Status(notifier=w917) -> (notifier out=w916:refnum<notifier>, current notification=w915:T11)  [unwired: 1 in, 3 out]
                n158 = Bundle By Name(cluster=w915, "Capture Exposure (s)"="Capture Exposure Time (s)", "Actions"=Orca_Flash_Capture_Actions."Idle") -> (w914:T11)
                n159 = Send Notification(notification=w914, notifier=w916) -> ()  [unwired: 1 in, 2 out]
              }
              frame "Email Address" {
                n160 = call "SMTP Email Alerts Messenger.vi"("Notifier Name"=w918, "Actions"=SMTP_Email_Alerts_Actions."Set Recipient", "Recipient"="Email Address") -> ()  [unwired: 13 in]
              }
            }
          }
          event "Live Preview", "Capture": Value Change {
            n161 = event-data() -> ("CtlRef"=w924:refnum<vi>, "NewVal"=w927:bool)  [unwired: 1 in]
            n162 = property class="Bool (strict)"(reference=w924) -> ("Label.Text"=w923:string)  [unwired: 1 in, 2 out]
            n163 = case shown="\"Live Preview\", Default" w923 {
              tunnel: [Orca_Flash_Capture_Actions."Capture" ("y") Orca_Flash_Capture_Actions."Live Preview" ("y")] -> w922
              frame "Capture" {
              }
              frame "Live Preview", Default {
              }
            }
            n164 = Select(t=w922, s=w927, f=Orca_Flash_Capture_Actions."Abort" ("y")) -> (s? t:f=w926:T12)
            n165 = Get Notifier Status(notifier=w929) -> (notifier out=w930:refnum<notifier>, current notification=w928:T11)  [unwired: 1 in, 3 out]
            n166 = Bundle By Name(cluster=w928, "Actions"=w926, "Running?"=w927) -> (w925:T11)
            n167 = Send Notification(notification=w925, notifier=w930) -> ()  [unwired: 1 in, 2 out]
          }
          event "Channels On/Off": Value Change {
            n168 = event-data() -> ("NewVal"=w950:bool)  [unwired: 1 in]
            n169 = Obtain Notifier(name (unnamed)="Display Module IMAQ Refs", notification data type=T7[] [], create if not found? (T)=FALSE) -> (notifier out=w943:refnum<notifier>, error out=w942:errorcluster)  [unwired: 1 in, 1 out]
            n170 = Get Notifier Status(notifier=w943, error in (no error)=w942) -> (notifier out=w941:refnum<notifier>, current notification=w939:T7[], error out=w940:errorcluster)  [unwired: 2 out]
            n171 = case shown="True" w950 {
              tunnel: w941 -> [w975 w991]
              tunnel: w940 -> [w974 w990]
              tunnel: [w971 w986] -> w946
              tunnel: [w975 w991] -> w947
              tunnel: [w974 w990] -> w945
              tunnel: w944 -> [w966 w989]
              tunnel: w939 -> [w973 w988]
              tunnel: w938 -> [w967 w985]
              tunnel: w937 -> [_ w984]
              tunnel: [w957 w984] -> w936
              tunnel: [T10."Enabled" ("Disabled") T10."Disabled and Grayed Out" ("Disabled")] -> w935
              frame False {
                n172 = control-ref of="This VI"() -> (w958:refnum<vi>)
                n173 = Equal?(x=w973, y=w967) -> (x = y?=w970:bool[])
                n174 = property class="VI"(reference=w958) -> (error out=w964:errorcluster, "Path"=w959:path)  [unwired: 1 in, 1 out]
                n175 = for {
                  tunnel: w970 -> [w982] mode=indexing
                  tunnel: [w981] -> w968
                  i -> [w981]
                  stop <- w982 stop-if-true
                }
                n176 = Or Array Elements(Boolean array=w970) -> (logical OR=w969:bool)
                n177 = Strip Path(path=w959) -> (stripped path=w963:path)  [unwired: 1 out]
                n178 = case shown="True" w969 {
                  tunnel: w968 -> [_ w979]
                  tunnel: w973 -> [w976 w978]
                  tunnel: [w976 w977] -> w972
                  frame False {
                  }
                  frame True {
                    n179 = Delete From Array(array=w978, length=1, index=w979) -> (array with subset deleted=w977:T7[])  [unwired: 1 out]
                  }
                }
                n180 = Build Path(base path=w963, name or relative path="ROI SubRegions.json") -> (appended path=w961:path)
                n181 = Read from Text File(file (use dialog)=w961, error in=w964) -> (text=w962:string, error out=w965:errorcluster)  [unwired: 2 in, 2 out]
                n182 = Build Array (concatenate)(w972, w966) -> (w971:T7[])
                n183 = Unflatten From JSON(JSON string=w962, type and defaults=T6[] [], error in (no error)=w965) -> (value=w957:T6[])  [unwired: 4 in, 1 out]
              }
              frame True {
                n184 = for {
                  tunnel: w989 -> [w994] mode=indexing
                  shift-right: [w992] -> w987
                  shift-left: w988 -> [w993]
                  n185 = Equal?(x=w993, y=w994) -> (x = y?=w997:bool[])
                  n186 = for {
                    tunnel: w997 -> [w1004] mode=indexing
                    tunnel: [w1003] -> w995
                    i -> [w1003]
                    stop <- w1004 stop-if-true
                  }
                  n187 = Or Array Elements(Boolean array=w997) -> (logical OR=w996:bool)
                  n188 = case shown="True" w996 {
                    tunnel: w995 -> [_ w1001]
                    tunnel: w993 -> [w998 w1000]
                    tunnel: [w998 w999] -> w992
                    frame False {
                    }
                    frame True {
                      n189 = Delete From Array(array=w1000, length=1, index=w1001) -> (array with subset deleted=w999:T7[])  [unwired: 1 out]
                    }
                  }
                }
                n190 = Build Array (concatenate)(w987, w985) -> (w986:T7[])
              }
            }
            n191 = Send Notification(notification=w946, notifier=w947, error in (no error)=w945) -> (notifier out=w949:refnum<notifier>, error out=w948:errorcluster)
            n192 = property on="Channel Array" class="Arr (strict)"("DisabledEnum"=w935) -> ()  [unwired: 2 in, 2 out]
            n193 = Release Notifier(notifier=w949, error in (no error)=w948) -> ()  [unwired: 1 in, 3 out]
          }
          event "Channel Array": Value Change {
            # "Remove all the image Refs from the array"
            n194 = event-data() -> ("NewVal"=w1013:T3[])  [unwired: 1 in]
            n195 = for {
              tunnel: w1013 -> [w1023] mode=indexing
              tunnel: w1014 -> [w1026] mode=indexing
              tunnel: [w1026] -> w1010 mode=indexing if=w1024
              tunnel: w1012 -> [w1025] mode=indexing
              tunnel: [w1022] -> w1011 mode=indexing
              n196 = Unbundle By Name(w1023) -> ("On/Off"=w1024:bool)
              n197 = Bundle By Name(cluster=w1025, "Active?"=w1024) -> (w1022:T6)
            }
            n198 = Obtain Notifier(name (unnamed)="Display Module IMAQ Refs", notification data type=T7[] [], create if not found? (T)=FALSE) -> (notifier out=w1017:refnum<notifier>, error out=w1016:errorcluster)  [unwired: 1 in, 1 out]
            n199 = Get Notifier Status(notifier=w1017, error in (no error)=w1016) -> (notifier out=w1005:refnum<notifier>, current notification=w1015:T7[])  [unwired: 3 out]
            n200 = for {
              tunnel: w1014 -> [w1032] mode=indexing
              shift-right: [w1027] -> w1009
              shift-left: w1015 -> [w1030]
              n201 = Search 1D Array(1D array=w1030, element=w1032, start index (0)=0) -> (index of element=w1029:i32)
              n202 = Delete From Array(array=w1030, length=1, index=w1029) -> (array with subset deleted=w1027:T7[])  [unwired: 1 out]
            }
            n203 = Build Array (concatenate)(w1010, w1009) -> (w1006:T7[])
            n204 = Send Notification(notification=w1006, notifier=w1005) -> (notifier out=w1008:refnum<notifier>, error out=w1007:errorcluster)  [unwired: 1 in]
            n205 = Release Notifier(notifier=w1008, error in (no error)=w1007) -> ()  [unwired: 1 in, 3 out]
          }
          event "Auto Update Subfolder": Value Change {
            n206 = event-data() -> ("NewVal"=w1037:bool)  [unwired: 1 in]
            n207 = Select(t=T10."Enabled" ("Disabled"), s=w1037, f=T10."Disabled and Grayed Out") -> (s? t:f=w1034:T10)
            n208 = property on="Subfolder Name" class="Str"("DisabledEnum"=w1034) -> ()  [unwired: 2 in, 2 out]
          }
          event "Line Scan Active": Value Change {
            n209 = event-data() -> ("NewVal"=w1039:bool)  [unwired: 1 in]
            n210 = Select(t="Frame Rate (Hz)", s=w1039, f="Exposure Time (s)") -> (s? t:f=w1060:string)
            n211 = Select(t=4.0, s=w1039, f=0.1) -> (s? t:f=w1053:dbl)
            n212 = Select(t=-1.0 ("f"), s=w1039, f=0.0) -> (s? t:f=w1044:dbl)
            n213 = Select(t=AO_SCTR_Actions."Update and Run" ("Actions"), s=w1039, f=AO_SCTR_Actions."Stop at Offset" ("Actions")) -> (s? t:f=w1045:T29)
            n214 = property on="Capture Exposure Time (s)" class="DigNum (strict)"("Caption.Text"=w1060, "Value"=w1053) -> ()  [unwired: 2 in, 2 out]
            n215 = property on="Preview Exposure Time (s)" class="DigNum (strict)"("Caption.Text"=w1060, "Value"=w1053) -> ()  [unwired: 2 in, 2 out]
            n216 = call "AO SCTR Messenger.vi"("Notifier Name"=w1041, "Actions"=w1045, "Offset (V)"=w1044) -> ()  [unwired: 12 in, 1 out]
            n217 = case shown="False" w1039 {
              frame False {
                w1064 = T10."Enabled" ("Disabled")
                n218 = property on="Preview Exposure Time (s)" class="DigNum (strict)"("DisabledEnum"=w1064) -> ()  [unwired: 2 in, 2 out]
                n219 = property on="Capture Exposure Time (s)" class="DigNum (strict)"("DisabledEnum"=w1064) -> ()  [unwired: 2 in, 2 out]
              }
              frame True {
              }
            }
            n220 = Get Notifier Status(notifier=w1057) -> (notifier out=w1056:refnum<notifier>, current notification=w1055:T11)  [unwired: 1 in, 3 out]
            n221 = Bundle By Name(cluster=w1055, "Line Scan?"=w1039, "Actions"=Orca_Flash_Capture_Actions."Idle", "Preview Exposure (s)"=w1053, "Capture Exposure (s)"=w1053) -> (w1052:T11)
            n222 = Select(t=Orca_Flash_Actions."PROGRESSIVE MODE" ("Camera Actions"), s=w1039, f=Orca_Flash_Actions."AREA MODE" ("Camera Actions")) -> (s? t:f=w1048:T21)
            n223 = call "Orca Flash Messanger.vi"("Notifier Name"=w1051, "Camera Actions"=w1048) -> ()  [unwired: 9 in, 5 out]
            n224 = Send Notification(notification=w1052, notifier=w1056) -> ()  [unwired: 1 in, 2 out]
          }
          event Value Change {
            n225 = event-data() -> ("NewVal"=w1074:T4)  [unwired: 1 in]
            n226 = Get Notifier Status(notifier=w1083) -> (notifier out=w1082:refnum<notifier>, current notification=w1081:T11)  [unwired: 1 in, 3 out]
            n227 = Bundle By Name(cluster=w1081, "Actions"=Orca_Flash_Capture_Actions."Idle", "Line Scan Mode"=w1074) -> (w1080:T11)
            n228 = Send Notification(notification=w1080, notifier=w1082) -> ()  [unwired: 1 in, 2 out]
            n229 = Equal?(x=w1074, y=Orca_Flash_Capture_Switch_Line_Scan_Modes."Use Presets") -> (x = y?=w1066:bool)
            n230 = Not Equal?(x=w1074, y=Orca_Flash_Capture_Switch_Line_Scan_Modes."Automatic") -> (x != y?=w1068:bool)
            n231 = Select(t=T10."Enabled" ("Disabled"), s=w1066, f=T10."Enabled" ("Disabled")) -> (s? t:f=w1076:T10)
            n232 = property on="Line Scanning Presets" class="Ring (strict)"("DisabledEnum"=w1076) -> ()  [unwired: 2 in, 2 out]
            n233 = case shown="True" w1066 {
              frame False {
              }
              frame True {
                n234 = property on="Line Scanning Presets" class="Ring (strict)"() -> ("Value"=w1086:u16)  [unwired: 2 in, 2 out]
                n235 = property on="Line Scanning Presets" class="Ring (strict)"("Val(Sgnl)"=w1086) -> ()  [unwired: 2 in, 2 out]
              }
            }
            n236 = Select(t=T10."Disabled and Grayed Out" ("Disabled"), s=w1068, f=T10."Enabled" ("Disabled")) -> (s? t:f=w1067:T10)
            n237 = Select(t=T10."Enabled" ("Disabled"), s=w1068, f=T10."Enabled" ("Disabled")) -> (s? t:f=w1071:T10)
            n238 = property on="Preview Exposure Time (s)" class="DigNum (strict)"("DisabledEnum"=w1067) -> ()  [unwired: 2 in, 2 out]
            n239 = property on="Capture Exposure Time (s)" class="DigNum (strict)"("DisabledEnum"=w1067) -> ()  [unwired: 2 in, 2 out]
            n240 = property on="Save As Preset" class="Bool"("DisabledEnum"=w1071) -> ()  [unwired: 2 in, 2 out]
            n241 = property on="Line Scan Settings" class="Clust (strict)"("DisabledEnum"=w1071) -> ()  [unwired: 2 in, 2 out]
          }
          event "Line Scanning Presets": Value Change {
            n242 = event-data() -> ("CtlRef"=w1096:refnum<vi>)  [unwired: 1 in]
            n243 = control-ref of="This VI"() -> (w1100:refnum<vi>)
            n244 = property class="Ring (strict)"(reference=w1096) -> ("RingText.Text"=w1094:string)  [unwired: 1 in, 2 out]
            n245 = property class="VI"(reference=w1100) -> ("Path"=w1099:path)  [unwired: 1 in, 2 out]
            n246 = Strip Path(path=w1099) -> (stripped path=w1098:path)  [unwired: 1 out]
            n247 = Concatenate Strings(w1094, ".json" ("string")) -> (w1092:string)
            n248 = Build Path(base path=w1098, name or relative path="Orca Flash Capture Manager Line Scan Presets") -> (appended path=w1095:path)
            n249 = Build Path(base path=w1095, name or relative path=w1092) -> (appended path=w1091:path)
            n250 = Read from Text File(file (use dialog)=w1091) -> (text=w1090:string, error out=w1088:errorcluster)  [unwired: 3 in, 2 out]
            n251 = Unflatten From JSON(JSON string=w1090, type and defaults=T5 {"Interline Interval"=0.0, "Offset (V)"=0.0, "Amplitude (V)"=0.0, "Samples Per Channel"=0.0, "Delay (ms)"=0.0} ("Line Scan Settings"), error in (no error)=w1088) -> (value=w1087:T5)  [unwired: 4 in, 1 out]
            n252 = property on="Line Scan Settings" class="Clust (strict)"("Val(Sgnl)"=w1087) -> ()  [unwired: 2 in, 2 out]
          }
          event Value Change {
            # "If you try and set the ILI while the camera is in area mode it gives an error"
            n253 = event-data() -> ("NewVal"=w1118:T5)  [unwired: 1 in]
            n254 = Get Notifier Status(notifier=w1123) -> (current notification=w1122:T11)  [unwired: 1 in, 4 out]
            n255 = Unbundle By Name(w1118) -> ("Offset (V)"=w1112:dbl, "Amplitude (V)"=w1116:dbl, "Samples Per Channel"=w1115:dbl, "Delay (ms)"=w1114:dbl, "Interline Interval"=w1107:dbl)
            n256 = Unbundle By Name(w1122) -> ("Line Scan?"=w1105:bool)
            n257 = To Long Integer(number=w1115) -> (32bit integer=w1113:i32)
            n258 = feedback-in #4(w1107) -> ()
            n259 = feedback #4(0.0) -> (w1106:dbl)
            n260 = Select(t=w1112, s=w1105, f=0.0) -> (s? t:f=w1110:dbl)
            n261 = Not Equal?(x=w1107, y=w1106) -> (x != y?=w1103:bool)
            n262 = Select(t=AO_SCTR_Actions."Update and Run" ("Actions"), s=w1105, f=AO_SCTR_Actions."Stop at Offset" ("Actions")) -> (s? t:f=w1119:T29)
            n263 = call "AO SCTR Messenger.vi"("Notifier Name"=w1117, "Actions"=w1119, "Offset (V)"=w1110, "Amplitude (V)"=w1116, "Samples Per Channel"=w1113, "Start Delay (ms)"=w1114) -> ()  [unwired: 9 in, 1 out]
            n264 = And(x=w1105, y=w1103) -> (x .and. y?=w1104:bool)
            n265 = case shown="True" w1104 {
              tunnel: w1109 -> [_ w1128]
              tunnel: w1107 -> [_ w1127]
              frame False {
              }
              frame True {
                n266 = Bundle By Name(cluster=T19 {"Value"=0.0, "Parameter"=4226016} ("sCMOS Parameter"), "Value"=w1127) -> (w1131:T19)
                n267 = call "Orca Flash Messanger.vi"("Notifier Name"=w1128, "Camera Actions"=Orca_Flash_Actions."SETPARAM", "sCMOS Parameter"=w1131) -> ("sCMOS Parameter"=w1132:T19)  [unwired: 8 in, 4 out]
                n268 = Unbundle By Name(w1132) -> ("Value"=w1126:dbl)
                n269 = property on="Interline Interval" class="DigNum (strict)"("Value"=w1126) -> ()  [unwired: 2 in, 2 out]
              }
            }
          }
          event "Save As Preset": Value Change {
            n270 = event-data() -> ()  [unwired: 1 in, 6 out]
            n271 = control-ref of="This VI"() -> (w1145:refnum<vi>)
            n272 = property class="VI"(reference=w1145) -> ("Path"=w1144:path)  [unwired: 1 in, 2 out]
            n273 = Strip Path(path=w1144) -> (stripped path=w1143:path)  [unwired: 1 out]
            n274 = Build Path(base path=w1143, name or relative path="Orca Flash Capture Manager Line Scan Presets") -> (appended path=w1134:path)
            n275 = call "File Dialog"("start path"=w1134, "prompt"="Save Preset File", "pattern (all files)"="*.json", "pattern label"="JSON") -> ("selected path"=w1139:path, "error out"=w1140:errorcluster)  [unwired: 8 in, 2 out]
            n276 = case shown="No Error" w1140 {
              selector: w1140 -> [_ w1165]
              tunnel: w1139 -> [w1164 _]
              tunnel: [w1158 w1165] -> w1133
              frame No Error {
                n277 = local read "Line Scan Settings"() -> (w1163:T5)
                n278 = Flatten To JSON(anything=w1163) -> (JSON string=w1162:string, 11:w1161:errorcluster)  [unwired: 2 in]
                n279 = Write to Text File(file (use dialog)=w1164, text=w1162, error in=w1161) -> (refnum out=w1160:refnum<file>, error out=w1159:errorcluster)  [unwired: 1 in, 1 out]
                n280 = Close File(refnum=w1160, error in=w1159) -> (error out=w1158:errorcluster)  [unwired: 1 out]
              }
              frame Error {
              }
            }
            n281 = List Folder(path=w1134, pattern="*.json", error in=w1133) -> (filenames=w1137:string[], error out=w1136:errorcluster)  [unwired: 1 in, 2 out]
            n282 = case shown="No Error" w1136 {
              tunnel: w1137 -> [w1152 _]
              tunnel: w1134 -> [w1151 _]
              tunnel: [w1150 string[] []] -> w1135
              frame No Error {
                n283 = for {
                  tunnel: w1152 -> [w1155] mode=indexing
                  tunnel: w1151 -> [w1156]
                  tunnel: [w1153] -> w1150 mode=indexing
                  n284 = Build Path(base path=w1156, name or relative path=w1155) -> (appended path=w1154:path)
                  n285 = call <vilib>:"Get File Extension.vi"("file"=w1154) -> ("filename without extension"=w1153:string)  [unwired: 6 in, 4 out]
                }
              }
              frame Error {
              }
            }
            n286 = property on="Line Scanning Presets" class="Ring (strict)"("Strings []"=w1135) -> ()  [unwired: 2 in, 2 out]
          }
          event "Edit Metadata": Value Change {
            n287 = event-data() -> ()  [unwired: 1 in, 1 out]
            n288 = call "Edit Sample Metadata.vi"() -> ()  [unwired: 14 in, 2 out]
          }
          event "Collect Metadata": Value Change {
            n289 = event-data() -> ("NewVal"=w1168:bool)  [unwired: 1 in]
            n290 = Get Notifier Status(notifier=w1170) -> (notifier out=w1173:refnum<notifier>, current notification=w1172:T11)  [unwired: 1 in, 3 out]
            n291 = Bundle By Name(cluster=w1172, "Actions"=Orca_Flash_Capture_Actions."Idle", "Collect Metadata?"=w1168) -> (w1171:T11)
            n292 = Send Notification(notification=w1171, notifier=w1173) -> ()  [unwired: 1 in, 2 out]
          }
          event "Quit": Value Change {
            n293 = event-data() -> ("NewVal"=w1190:bool)  [unwired: 1 in]
            n294 = Get Notifier Status(notifier=w1189) -> (notifier out=w1188:refnum<notifier>, current notification=w1187:T11)  [unwired: 1 in, 3 out]
            n295 = Bundle By Name(cluster=w1187, "Running?"=FALSE ("Abort"), "Actions"=Orca_Flash_Capture_Actions."Quit") -> (w1181:T11)
            n296 = Send Notification(notification=w1181, notifier=w1188) -> (notifier out=w1185:refnum<notifier>)  [unwired: 1 in, 1 out]
            n297 = Wait on Notification(notifier=w1185, ignore previous (F)=TRUE, timeout in ms (-1)=500) -> (notifier out=w1182:refnum<notifier>)  [unwired: 1 in, 3 out]
            n298 = Send Notification(notification=w1181, notifier=w1182) -> (notifier out=w1179:refnum<notifier>)  [unwired: 1 in, 1 out]
            n299 = Release Notifier(notifier=w1179, force destroy? (F)=TRUE) -> ()  [unwired: 1 in, 3 out]
            n300 = for {
              tunnel: w1177 -> [w1191] mode=indexing
              n301 = call "IMAQ Dispose"("Image"=w1191) -> ()  [unwired: 5 in, 1 out]
            }
          }
        }
      }
      n302 = while {
        tunnel: w241 -> [w272]
        tunnel: w209 -> [w266]
        tunnel: w240 -> [w264]
        tunnel: [FALSE] -> w239
        tunnel: w233 -> [w262]
        tunnel: w203 -> [w260]
        tunnel: w202 -> [w259]
        tunnel: w201 -> [w258]
        tunnel: w200 -> [w257]
        tunnel: [w257] -> w199
        tunnel: w192 -> [w256]
        tunnel: w191 -> [w252]
        tunnel: [w252] -> w190
        stop <- w268 stop-if-true
        w254 = u16 0 ("Current Step")
        n303 = Wait on Notification(notifier=w272, ignore previous (F)=TRUE) -> (notifier out=w267:refnum<notifier>, notification=w270:T11)  [unwired: 2 in, 2 out]
        n304 = Unbundle By Name(w270) -> ("Actions"=w265:T12)
        n305 = Bundle By Name(cluster=T22 {"Scan Mode"=enum."Steps Then Cycles", "Current Step"=0, "Current Cycle"=0, "Num of Steps"=0, "Num of Cycles"=0} ("Cycles Steps Tracker"), "Current Step"=w254, "Current Cycle"=w254, "Num of Steps"=w254, "Num of Cycles"=w254, "Scan Mode"="Scan Mode") -> (w261:T22)
        n306 = Equal?(x=w265, y=Orca_Flash_Capture_Actions."Quit") -> (x = y?=w268:bool)
        n307 = while {
          shift-right: [w288] -> _
          shift-left: w265 -> [w289]
          tunnel: w267 -> [w282]
          tunnel: w266 -> [w285]
          tunnel: w265 -> [w284]
          tunnel: w264 -> [w283]
          tunnel: w262 -> [w281]
          shift-right: [w279] -> _
          shift-left: w261 -> [w280]
          tunnel: w260 -> [w278]
          tunnel: w259 -> [w277]
          tunnel: w258 -> [w276]
          tunnel: w257 -> [w275]
          tunnel: w256 -> [w274]
          tunnel: w252 -> [w273]
          stop <- w286 stop-if-true
          n308 = case shown="\"Write Metadata\"" w289 {
            selector: w289 -> [_ _ _ w370 _ _ _ _ _ _ _ _ _ _ _]
            tunnel: [Orca_Flash_Capture_Actions."Quit" ("y") Orca_Flash_Capture_Actions."Laser On" ("y") Orca_Flash_Capture_Actions."Laser Off" ("y") w364 Orca_Flash_Capture_Actions."Start Acquisition" ("y") w435 Orca_Flash_Capture_Actions."Write Metadata" ("y") w533 Orca_Flash_Capture_Actions."Camera" ("y") w575 w613 Orca_Flash_Capture_Actions."Setup" ("y") Orca_Flash_Capture_Actions."External Cycle Sync" ("y") w736 Orca_Flash_Capture_Actions."Quit" ("y")] -> w288
            tunnel: [w291 w303 w333 w368 w392 w437 w504 w541 w553 w583 w633 w648 w704 w757 TRUE] -> w286
            tunnel: FALSE -> [w291 w303 w333 w368 w392 w437 w504 w541 w553 w583 w633 w648 w704 w757 _]
            tunnel: w285 -> [_ w296 w330 _ w377 w436 _ _ _ w572 _ _ _ _ _]
            tunnel: w284 -> [_ _ w329 _ w385 w433 w501 w539 _ _ _ _ _ _ _]
            tunnel: w283 -> [_ _ _ w367 _ _ _ _ _ _ _ _ _ _ _]
            tunnel: w282 -> [_ _ w327 _ w390 w434 w503 w532 _ w576 w620 w640 w702 _ w779]
            tunnel: w281 -> [_ _ w324 _ _ w432 _ _ _ _ _ w639 w703 _ _]
            tunnel: w280 -> [w290 w302 w310 w362 w380 w431 w502 w540 w551 w568 w618 w638 w687 w756 w789]
            tunnel: [w290 w302 w310 w362 w380 w430 w502 w540 w551 w568 w632 w638 w687 w756 w789] -> w279
            tunnel: w278 -> [_ _ _ _ w373 _ _ _ _ _ _ _ _ _ _]
            tunnel: w277 -> [_ _ _ _ w372 _ _ _ _ _ _ _ _ _ _]
            tunnel: w276 -> [_ _ _ _ w371 _ _ _ _ _ _ _ _ _ _]
            tunnel: w275 -> [_ w295 _ _ _ w429 _ _ _ w567 _ _ w688 _ w784]
            tunnel: w274 -> [_ _ w306 _ _ _ _ _ _ _ _ _ _ _ _]
            tunnel: w273 -> [_ _ _ _ _ _ _ _ _ w555 _ _ _ _ _]
            frame "Idle", Default {
            }
            frame "Live Preview", "Capture" {
              w293 = FALSE ("Camera Running?")
              n309 = call "Orca Flash Messanger.vi"("Notifier Name"=w296, "Camera Actions"=Orca_Flash_Actions."STATUS") -> ("Image Ref"=w297:T7)  [unwired: 9 in, 4 out]
              n310 = Get Notifier Status(notifier=w295) -> (notifier out=w300:refnum<notifier>, current notification=w301:T8)  [unwired: 1 in, 3 out]
              n311 = Bundle By Name(cluster=w301, "Image Ref"=w297, "Cycle Number"=u16 0, "Camera Running?"=w293, "Capture?"=w293) -> (w299:T8)
              n312 = Send Notification(notification=w299, notifier=w300) -> ()  [unwired: 1 in, 2 out]
            }
            frame "Abort" {
              w326 = u16 1 ("Current Cycle")
              w331 = FALSE ("Live Preview")
              n313 = call "Orca Flash Messanger.vi"("Notifier Name"=w330, "Camera Actions"=Orca_Flash_Actions."IDLE") -> ()  [unwired: 9 in, 5 out]
              n314 = local write "Live Preview"(w331) -> ()
              n315 = local write "Capture"(w331) -> ()
              n316 = Equal?(x=Orca_Flash_Capture_Actions."Capture", y=w329) -> (x = y?=w323:bool)
              n317 = Get Notifier Status(notifier=w327) -> (current notification=w305:T11)  [unwired: 1 in, 4 out]
              n318 = local write "Current Cycle"(w326) -> ()
              n319 = local write "Current Step"(w326) -> ()
              n320 = Unbundle By Name(w305) -> ("Init Z Position (µm)"=w325:dbl)
              n321 = Obtain Notifier(name (unnamed)="WFDC External Sync", notification data type=T24 {"Cycle Sync"=enum."Pause Requested", "Z Offset"=0.0, "WFDC Status"=enum."Idle"} ("WFDC External Sync"), create if not found? (T)=FALSE) -> (notifier out=w317:refnum<notifier>, error out=w322:errorcluster)  [unwired: 1 in, 1 out]
              n322 = Get Notifier Status(notifier=w317, error in (no error)=w322) -> (notifier out=w312:refnum<notifier>, current notification=w311:T24, error out=w321:errorcluster)  [unwired: 2 out]
              n323 = Unbundle By Name(w311) -> ("WFDC Status"=w309:T23)
              n324 = Unbundle By Name(w321) -> ("status"=w320:bool)
              n325 = Not Equal?(x=WFDC_Status."DC Active", y=w309) -> (x != y?=w319:bool)
              n326 = Equal?(x=w309, y=WFDC_Status."Error") -> (x = y?=w307:bool)
              n327 = Or(x=w319, y=w320) -> (x .or. y?=w313:bool)
              n328 = case shown="True" w323 {
                tunnel: w325 -> [_ w342]
                tunnel: w324 -> [_ w341]
                tunnel: w313 -> [_ w340]
                tunnel: w312 -> [_ w339]
                tunnel: w311 -> [_ w338]
                tunnel: w307 -> [_ w336]
                tunnel: w306 -> [_ w335]
                frame False {
                }
                frame True {
                  n329 = case shown="True" w340 {
                    tunnel: w342 -> [_ w360]
                    tunnel: w341 -> [_ w359]
                    tunnel: w339 -> [w353 _]
                    tunnel: w338 -> [w352 _]
                    frame False {
                      n330 = Bundle By Name(cluster=w352, "Z Offset"=0.0) -> (w354:T24)
                      n331 = Send Notification(notification=w354, notifier=w353) -> (notifier out=w349:refnum<notifier>)  [unwired: 1 in, 1 out]
                      n332 = Release Notifier(notifier=w349, force destroy? (F)=FALSE) -> ()  [unwired: 1 in, 3 out]
                    }
                    frame True {
                      n333 = Build Array(w360) -> (w355:dbl[])
                      n334 = call "Stages Messenger.vi"("Stage Notifier Name"=w359, "Actions"=Stage_Actions."MOVE", "Setpoint"=w355, "Axis"=bool[] [TRUE], "Exit While Busy?"=FALSE) -> ()  [unwired: 7 in, 4 out]
                    }
                  }
                  n335 = case shown="True" "Email Alerts" {
                    tunnel: w336 -> [_ w345]
                    tunnel: w335 -> [_ w343]
                    frame False {
                    }
                    frame True {
                      n336 = Select(t="Acquisition Error - Abort", s=w345, f="Acquisition Finished") -> (s? t:f=w344:string)
                      n337 = call "SMTP Email Alerts Messenger.vi"("Notifier Name"=w343, "Actions"=SMTP_Email_Alerts_Actions."Send Message", "Subject"=w344, "Body Text"=w344) -> ()  [unwired: 12 in]
                    }
                  }
                }
              }
            }
            frame "Laser On", "Laser Off" {
              n338 = Equal?(x=w370, y=Orca_Flash_Capture_Actions."Laser On") -> (x = y?=w361:bool)
              n339 = call "AOTF Messenger.vi"("AOTF Notifier Name"=w367, "AOTF Action"=AOTF_Actions."Blank", "Beam Blank"=w361) -> ()  [unwired: 7 in, 6 out]
              n340 = Select(t=Orca_Flash_Capture_Actions."Set Exposure Time" ("y"), s=w361, f=Orca_Flash_Capture_Actions."Quit" ("y")) -> (s? t:f=w364:T12)
            }
            frame "Set Exposure Time" {
              # "Frame Rate (Hz)"
              n341 = Get Notifier Status(notifier=w390) -> (current notification=w386:T11)  [unwired: 1 in, 4 out]
              n342 = Unbundle By Name(w386) -> ("Line Scan?"=w375:bool, "Line Scan Mode"=w374:T4, "Capture Exposure (s)"=w381:dbl, "Preview Exposure (s)"=w382:dbl)
              n343 = Equal?(x=w385, y=Orca_Flash_Capture_Actions."Capture") -> (x = y?=w383:bool)
              n344 = Select(t=w381, s=w383, f=w382) -> (s? t:f=w379:dbl)
              n345 = case shown="True" w375 {
                tunnel: w379 -> [w394 w403]
                tunnel: [w394 w400] -> w378
                tunnel: w377 -> [w393 w402]
                tunnel: [w393 w399] -> w376
                tunnel: w374 -> [_ w398]
                tunnel: w373 -> [_ w397]
                tunnel: w372 -> [_ w396]
                tunnel: w371 -> [_ w395]
                frame False {
                  # "Exposure Time (s)"
                }
                frame True {
                  n346 = To Double Precision Float(number="Number of Lines") -> (double precision float=w401:dbl)
                  n347 = case shown="\"Automatic\"" w398 {
                    tunnel: w403 -> [_ w428]
                    tunnel: w402 -> [w409 w427]
                    tunnel: w401 -> [w407 w426]
                    tunnel: [w405 w425] -> w400
                    tunnel: [w408 w424] -> w399
                    tunnel: w397 -> [_ w417]
                    tunnel: w396 -> [_ w414]
                    tunnel: w395 -> [_ w413]
                    frame Default {
                      n348 = call "Orca Flash Messanger.vi"("Notifier Name"=w409, "Camera Actions"=Orca_Flash_Actions."GETPARAM", "sCMOS Parameter"=T19 {"Value"=0.0, "Parameter"=4226016}) -> ("Notifier Name Dup"=w408:string, "sCMOS Parameter"=w412:T19)  [unwired: 8 in, 3 out]
                      n349 = Unbundle By Name(w412) -> ("Value"=w406:dbl)
                      n350 = Multiply(x=w406, y=w407) -> (x*y=w405:dbl)
                    }
                    frame "Automatic" {
                      n351 = call "Orca Flash Capture Set Interline Interval.vi"("Camera Notifier Name"=w427, "Frame Rate (Hz)"=w428) -> ("Camera Notifier Name (Dup)"=w424:string, "Interline Interval (s)"=w423:dbl)  [unwired: 12 in]
                      n352 = Multiply(x=w423, y=w426) -> (x*y=w425:dbl)
                      n353 = call "Orca Flash Capture Set Auto Waveform.vi"("Interline Interval"=w423, "Filter Index"="Current Filter", "Waveform Parameters"=w414, "Filter Offsets"=w413) -> ("Offset (V)"=w421:dbl, "Amplitude (V)"=w420:dbl, "Samples per Channel"=w419:i32, "Delay (ms)"=w418:dbl, "Line Scan Settings"=w416:T5)  [unwired: 7 in]
                      n354 = local write "Line Scan Settings"(w416) -> ()
                      n355 = call "AO SCTR Messenger.vi"("Notifier Name"=w417, "Actions"=AO_SCTR_Actions."Update and Run", "Offset (V)"=w421, "Amplitude (V)"=w420, "Samples Per Channel"=w419, "Start Delay (ms)"=w418) -> ()  [unwired: 9 in, 1 out]
                    }
                  }
                }
              }
              n356 = Bundle By Name(cluster=T19 {"Value"=0.0, "Parameter"=2049184} ("sCMOS Parameter"), "Value"=w378) -> (w389:T19)
              n357 = call "Orca Flash Messanger.vi"("Notifier Name"=w376, "Camera Actions"=Orca_Flash_Actions."SETPARAM", "sCMOS Parameter"=w389) -> ()  [unwired: 8 in, 5 out]
            }
            frame "Start Acquisition" {
              n358 = case shown="\"Capture\"" w433 {
                tunnel: w436 -> [_ w440 _]
                tunnel: [Orca_Flash_Capture_Actions."Quit" ("y") Orca_Flash_Capture_Actions."Quit" ("y") Orca_Flash_Capture_Actions."Update SubFolder" ("y")] -> w435
                tunnel: w434 -> [_ _ w475]
                tunnel: w432 -> [_ _ w467]
                tunnel: w431 -> [w438 w441 w463]
                tunnel: [w438 w441 w462] -> w430
                tunnel: w429 -> [_ _ w455]
                frame Default {
                }
                frame "Live Preview" {
                  n359 = call "Orca Flash Messanger.vi"("Notifier Name"=w440, "Camera Actions"=Orca_Flash_Actions."PREVIEW") -> ()  [unwired: 9 in, 5 out]
                }
                frame "Capture" {
                  w461 = sgl 0.0 ("Cycle")
                  n360 = Get Notifier Status(notifier=w455) -> (notifier out=w459:refnum<notifier>, current notification=w458:T8)  [unwired: 1 in, 3 out]
                  n361 = Bundle By Name(cluster=w458, "Capture?"=TRUE) -> (w457:T8)
                  n362 = call "Stages Messenger.vi"("Stage Notifier Name"=w467, "Actions"=Stage_Actions."Get Position") -> ("Positions"=w470:dbl[])  [unwired: 10 in, 3 out]
                  n363 = Send Notification(notification=w457, notifier=w459) -> ()  [unwired: 1 in, 2 out]
                  n364 = Index Array(array=w470, index=0) -> (element=w468:dbl)
                  n365 = local write "Z Step"(w461) -> ()
                  n366 = local write "Cycle"(w461) -> ()
                  n367 = local write "Frame"(u32 0 ("Frame")) -> ()
                  n368 = Get Notifier Status(notifier=w475) -> (notifier out=w472:refnum<notifier>, current notification=w473:T11)  [unwired: 1 in, 3 out]
                  n369 = Bundle By Name(cluster=w473, "Init Z Position (µm)"=w468) -> (w464:T11)
                  n370 = Unbundle By Name(w464) -> ("Cycles"=w465:u16, "No. of Z Steps"=w466:u16)
                  n371 = Send Notification(notification=w464, notifier=w472) -> ()  [unwired: 1 in, 2 out]
                  n372 = Bundle By Name(cluster=w463, "Num of Cycles"=w465, "Num of Steps"=w466) -> (w462:T22)
                  n373 = Obtain Notifier(name (unnamed)="WFDC External Sync", notification data type=T24 {"Cycle Sync"=enum."Pause Requested", "Z Offset"=0.0, "WFDC Status"=enum."Idle"} ("WFDC External Sync"), create if not found? (T)=FALSE) -> (notifier out=w453:refnum<notifier>, error out=w454:errorcluster)  [unwired: 1 in, 1 out]
                  n374 = Get Notifier Status(notifier=w453, error in (no error)=w454) -> (notifier out=w448:refnum<notifier>, current notification=w447:T24, error out=w446:errorcluster)  [unwired: 2 out]
                  n375 = Unbundle By Name(w447) -> ("WFDC Status"=w449:T23)
                  n376 = case shown="\"Error\"" w449 {
                    tunnel: w448 -> [w478 w483]
                    tunnel: w447 -> [_ w482]
                    tunnel: w446 -> [w477 w480]
                    tunnel: [w478 w481] -> w444
                    tunnel: [w477 w479] -> w445
                    frame Default {
                    }
                    frame "Error" {
                      n377 = Two Button Dialog(message="Reset Wide Field Drift Correction error?", 1:"No" ("F button name (\"Cancel\")"), 2:"Yes" ("T button name (\"OK\")")) -> (T button?=w487:bool)
                      n378 = case shown="True" w487 {
                        tunnel: w483 -> [w489 w494]
                        tunnel: w482 -> [_ w496]
                        tunnel: [w489 w492] -> w481
                        tunnel: w480 -> [w488 w491]
                        tunnel: [w488 w490] -> w479
                        frame False {
                        }
                        frame True {
                          n379 = Bundle By Name(cluster=w496, "WFDC Status"=WFDC_Status."Idle") -> (w493:T24)
                          n380 = Send Notification(notification=w493, notifier=w494, error in (no error)=w491) -> (notifier out=w492:refnum<notifier>, error out=w490:errorcluster)
                        }
                      }
                    }
                  }
                  n381 = case shown="No Error" w445 {
                    tunnel: w444 -> [w476 _]
                    frame No Error {
                      n382 = Release Notifier(notifier=w476) -> ()  [unwired: 2 in, 3 out]
                    }
                    frame Error {
                    }
                  }
                }
              }
            }
            frame "Update SubFolder" {
              n383 = Equal?(x=w501, y=Orca_Flash_Capture_Actions."Capture") -> (x = y?=w499:bool)
              n384 = And(x=w499, y="Auto Update Subfolder") -> (x .and. y?=w497:bool)
              n385 = case shown="True" w497 {
                tunnel: w503 -> [w510 w526]
                frame False {
                  n386 = Get Notifier Status(notifier=w510) -> (notifier out=w509:refnum<notifier>, current notification=w507:T11)  [unwired: 1 in, 3 out]
                  n387 = Unbundle By Name(w507) -> ("Base Path"=w506:path)
                  n388 = Bundle By Name(cluster=w507, "Save Path"=w506) -> (w508:T11)
                  n389 = Send Notification(notification=w508, notifier=w509) -> ()  [unwired: 1 in, 2 out]
                }
                frame True {
                  n390 = Get Notifier Status(notifier=w526) -> (notifier out=w514:refnum<notifier>, current notification=w513:T11)  [unwired: 1 in, 3 out]
                  n391 = feedback #5(u32 0) -> (w516:u32)
                  n392 = Unbundle By Name(w513) -> ("Base Path"=w525:path)
                  n393 = Increment(x=w516) -> (x+1=w515:u32)
                  n394 = feedback-in #5(w515) -> ()
                  n395 = Format Into String(format string="%03d", w515) -> (resulting string=w517:string)  [unwired: 2 in, 1 out]
                  n396 = Strip Path(path=w525) -> (stripped path=w524:path, name=w522:string)
                  n397 = Concatenate Strings("Subfolder Name", w517) -> (w520:string)
                  n398 = Build Path(base path=w524, name or relative path=w520) -> (appended path=w523:path)
                  n399 = Build Path(base path=w523, name or relative path=w522) -> (appended path=w512:path)
                  n400 = Bundle By Name(cluster=w513, "Save Path"=w512) -> (w511:T11)
                  n401 = Send Notification(notification=w511, notifier=w514) -> ()  [unwired: 1 in, 2 out]
                }
              }
            }
            frame "Write Metadata" {
              n402 = Get Notifier Status(notifier=w532) -> (notifier out=w531:refnum<notifier>, current notification=w530:T11)  [unwired: 1 in, 3 out]
              n403 = Unbundle By Name(w530) -> ("Collect Metadata?"=w527:bool)
              n404 = Equal?(x=w539, y=Orca_Flash_Capture_Actions."Capture") -> (x = y?=w529:bool)
              n405 = And(x=w527, y=w529) -> (x .and. y?=w528:bool)
              n406 = case shown="True" w528 {
                tunnel: w531 -> [_ w550]
                tunnel: [errorcluster {"status"=FALSE, "code"=0, "source"=""} ("Write Errror") w543] -> w537
                frame False {
                }
                frame True {
                  n407 = Get Notifier Status(notifier=w550) -> (current notification=w549:T11)  [unwired: 1 in, 4 out]
                  n408 = Unbundle By Name(w549) -> ("Save Path"=w548:path)
                  n409 = call "Write Device Metadata.vi"("File Path"=w548) -> ("File Path (Dup)"=w547:path, "Write Errror"=w546:errorcluster)  [unwired: 13 in]
                  n410 = call "Write Microscope Metadata.vi"("File Path"=w547, "Error In"=w546) -> ("File Path (Dup)"=w544:path, "Write Errror"=w545:errorcluster)  [unwired: 12 in]
                  n411 = call "Run Sample Metadata.vi"("Image File (Path/Name)"=w544, "Error In"=w545) -> ("Error Out"=w543:errorcluster)  [unwired: 12 in, 1 out]
                }
              }
              n412 = Unbundle By Name(w537) -> ("status"=w536:bool)
              n413 = Select(t=Orca_Flash_Capture_Actions."Abort" ("y"), s=w536, f=Orca_Flash_Capture_Actions."Setup" ("y")) -> (s? t:f=w533:T12)
            }
            frame "Setup" {
              # "Change lasers here"
            }
            frame "Camera" {
              n414 = Get Notifier Status(notifier=w576) -> (notifier out=w582:refnum<notifier>, current notification=w569:T11)  [unwired: 1 in, 3 out]
              n415 = Unbundle By Name(w568) -> ("Current Cycle"=w574:u16, "Current Step"=w573:u16)
              n416 = Unbundle By Name(w569) -> ("Save Path"=w579:path, "Frames"=w570:u32)
              n417 = call "Orca Flash Capture File Name Increment.vi"("Path In"=w579, "Cycle"=w574, "Step"=w573) -> ("Path Out"=w556:path)  [unwired: 12 in]
              n418 = Get Notifier Status(notifier=w567) -> (notifier out=w566:refnum<notifier>, current notification=w565:T8)  [unwired: 1 in, 3 out]
              n419 = Bundle By Name(cluster=w565, "Camera Running?"=TRUE) -> (w563:T8)
              n420 = call "Orca Flash Messanger.vi"("Notifier Name"=w572, "Camera Actions"=Orca_Flash_Actions."Record Settings", "Path"=w556, "# of frames"=w570) -> ("Notifier Name Dup"=w581:string)  [unwired: 7 in, 4 out]
              n421 = call "Orca Flash Messanger.vi"("Notifier Name"=w581, "Camera Actions"=Orca_Flash_Actions."RECORD") -> ("Notifier Name Dup"=w577:string, "Image Ref"=w571:T7)  [unwired: 9 in, 3 out]
              n422 = Send Notification(notification=w563, notifier=w566) -> (notifier out=w562:refnum<notifier>)  [unwired: 1 in, 1 out]
              n423 = while {
                tunnel: w577 -> [w606]
                tunnel: [w603] -> w575
                tunnel: w582 -> [w592]
                tunnel: w571 -> [w591]
                tunnel: [w585] -> w558
                tunnel: w562 -> [w585]
                tunnel: w556 -> [w584]
                tunnel: [w584] -> w554
                stop <- w599 stop-if-true
                n424 = Get Notifier Status(notifier=w592) -> (current notification=w605:T11)  [unwired: 1 in, 4 out]
                n425 = Unbundle By Name(w605) -> ("Running?"=w598:bool)
                n426 = Wait (ms)(milliseconds to wait=u32 25) -> ()  [unwired: 1 out]
                n427 = call "IMAQ Read Custom Data"("Key"="Image Data", "Image"=w591) -> ("Custom Data Out"=w589:string)  [unwired: 7 in, 2 out]
                n428 = Unflatten From JSON(JSON string=w589, type and defaults=T30 {"Frame"=0, "Sensor Height"=0, "Sensor Width"=0, "ROI Height"=0, "ROI Width"=0, "ROI Enable?"=FALSE, "Bit per Pixel"=0} ("Camera IMAQ Key Info")) -> (value=w587:T30)  [unwired: 5 in, 1 out]
                n429 = Not(x=w598) -> (.not. x?=w602:bool)
                n430 = Unbundle By Name(w587) -> ("Frame"=→"Frame" →"Current Frame":u32)
                n431 = Select(t=Orca_Flash_Actions."STATUS" ("Camera Actions"), s=w598, f=Orca_Flash_Actions."IDLE") -> (s? t:f=w593:T21)
                n432 = call "Orca Flash Messanger.vi"("Notifier Name"=w606, "Camera Actions"=w593) -> ("Running?"=w601:bool)  [unwired: 9 in, 4 out]
                n433 = Not(x=w601) -> (.not. x?=w600:bool)
                n434 = Or(x=w602, y=w600) -> (x .or. y?=w599:bool)
                n435 = Select(t=Orca_Flash_Capture_Actions."Switch" ("y"), s=w598, f=Orca_Flash_Capture_Actions."Abort") -> (s? t:f=w603:T12)
              }
              n436 = Get Notifier Status(notifier=w558) -> (notifier out=w557:refnum<notifier>, current notification=w559:T8)  [unwired: 1 in, 3 out]
              n437 = Bundle By Name(cluster=w559, "Camera Running?"=FALSE) -> (w561:T8)
              n438 = Send Notification(notification=w561, notifier=w557) -> ()  [unwired: 1 in, 2 out]
              n439 = Enqueue Element(queue=w555, element=w554) -> ()  [unwired: 2 in, 3 out]
            }
            frame "Switch" {
              n440 = Get Notifier Status(notifier=w620) -> (current notification=w619:T11)  [unwired: 1 in, 4 out]
              n441 = Unbundle By Name(w619) -> ("Cycles"=w615:u16, "No. of Z Steps"=w616:u16)
              n442 = Bundle By Name(cluster=w618, "Num of Cycles"=w615, "Num of Steps"=w616) -> (w617:T22)
              n443 = Unbundle By Name(w617) -> ("Current Cycle"=w629:u16, "Num of Cycles"=w628:u16, "Current Step"=w627:u16, "Num of Steps"=w626:u16)
              n444 = Increment(x=w629) -> (x+1=w612:u16)
              n445 = Increment(x=w627) -> (x+1=w611:u16)
              n446 = To Single Precision Float(number=w612) -> (single precision float=w625:sgl)
              n447 = To Single Precision Float(number=w628) -> (single precision float=w624:sgl)
              n448 = To Single Precision Float(number=w611) -> (single precision float=w623:sgl)
              n449 = To Single Precision Float(number=w626) -> (single precision float=w622:sgl)
              n450 = Divide(x=w625, y=w624) -> (x/y=→"Cycle":sgl)
              n451 = Divide(x=w623, y=w622) -> (x/y=→"Z Step":sgl)
              n452 = call "Orca Flash Capture Scan Counter Cycles Steps.vi"("Cycles Steps Tracker"=w617) -> ("Cycles Steps Tracker Out"=w632:T22, "Change Cycle?"=w609:bool, "Done?"=w631:bool)  [unwired: 8 in]
              n453 = Select(t=Orca_Flash_Capture_Actions."Cycle" ("y"), s=w609, f=Orca_Flash_Capture_Actions."Step") -> (s? t:f=w607:T12)
              n454 = Select(t=Orca_Flash_Capture_Actions."Abort" ("y"), s=w631, f=w607) -> (s? t:f=w613:T12)
              n455 = case shown="Default" w613 {
                tunnel: w612 -> [_ w635 _]
                tunnel: w611 -> [_ _ w637]
                frame Default {
                }
                frame "Cycle" {
                  n456 = Increment(x=w635) -> (x+1=→"Current Cycle":u16)
                }
                frame "Step" {
                  n457 = Increment(x=w637) -> (x+1=→"Current Step":u16)
                }
              }
            }
            frame "Step" {
              n458 = Get Notifier Status(notifier=w640) -> (current notification=w641:T11)  [unwired: 1 in, 4 out]
              n459 = Unbundle By Name(w641) -> ("Z Step Size (µm)"=w647:dbl, "No. of Z Steps"=w644:u16)
              n460 = Less?(x=w644, y=u16 2) -> (x < y?=w645:bool)
              n461 = Equal To 0?(x=w647) -> (x = 0?=w642:bool)
              n462 = Or(x=w642, y=w645) -> (x .or. y?=w643:bool)
              n463 = case shown="False" w643 {
                tunnel: w639 -> [w667 _]
                tunnel: w647 -> [w666 _]
                tunnel: w638 -> [w653 _]
                frame False {
                  n464 = Unbundle By Name(w653) -> ("Current Step"=w652:u16)
                  n465 = Obtain Notifier(name (unnamed)="WFDC External Sync", notification data type=T24 {"Cycle Sync"=enum."Pause Requested", "Z Offset"=0.0, "WFDC Status"=enum."Idle"} ("WFDC External Sync"), create if not found? (T)=FALSE) -> (notifier out=w659:refnum<notifier>, error out=w665:errorcluster)  [unwired: 1 in, 1 out]
                  n466 = Get Notifier Status(notifier=w659, error in (no error)=w665) -> (notifier out=w654:refnum<notifier>, current notification=w651:T24, error out=w664:errorcluster)  [unwired: 2 out]
                  n467 = Unbundle By Name(w651) -> ("WFDC Status"=w660:T23)
                  n468 = Unbundle By Name(w664) -> ("status"=w663:bool)
                  n469 = Not Equal?(x=WFDC_Status."DC Active", y=w660) -> (x != y?=w662:bool)
                  n470 = Or(x=w662, y=w663) -> (x .or. y?=w655:bool)
                  n471 = case shown="False" w655 {
                    tunnel: w667 -> [_ w683]
                    tunnel: w666 -> [w674 w682]
                    tunnel: w654 -> [w671 _]
                    tunnel: w652 -> [w676 _]
                    tunnel: w651 -> [w675 _]
                    tunnel: [u32 350 ("milliseconds to wait") u32 100 ("milliseconds to wait")] -> w650
                    frame False {
                      n472 = To Double Precision Float(number=w676) -> (double precision float=w673:dbl)
                      n473 = Multiply(x=w674, y=w673) -> (x*y=w672:dbl)
                      n474 = Bundle By Name(cluster=w675, "Z Offset"=w672) -> (w670:T24)
                      n475 = Send Notification(notification=w670, notifier=w671) -> (notifier out=w668:refnum<notifier>)  [unwired: 1 in, 1 out]
                      n476 = Release Notifier(notifier=w668) -> ()  [unwired: 2 in, 3 out]
                    }
                    frame True {
                      n477 = Build Array(w682) -> (w681:dbl[])
                      n478 = call "Stages Messenger.vi"("Stage Notifier Name"=w683, "Actions"=Stage_Actions."MVR", "Setpoint"=w681, "Axis"=bool[] [TRUE], "Exit While Busy?"=FALSE) -> ()  [unwired: 7 in, 4 out]
                    }
                  }
                  n479 = Wait (ms)(milliseconds to wait=w650) -> ()  [unwired: 1 out]
                }
                frame True {
                }
              }
            }
            frame "Cycle" {
              n480 = Unbundle By Name(w687) -> ("Scan Mode"=w686:T2, "Current Cycle"=w689:u16)
              n481 = Equal?(x=Orca_Flash_Switch_Cycles_Steps."Cycles Then Steps", y=w686) -> (x = y?=w684:bool)
              n482 = Get Notifier Status(notifier=w702) -> (current notification=w701:T11)  [unwired: 1 in, 4 out]
              n483 = Get Notifier Status(notifier=w688) -> (notifier out=w692:refnum<notifier>, current notification=w691:T8)  [unwired: 1 in, 3 out]
              n484 = Bundle By Name(cluster=w691, "Cycle Number"=w689) -> (w690:T8)
              n485 = Unbundle By Name(w701) -> ("Init Z Position (µm)"=w693:dbl, "Z Step Size (µm)"=w697:dbl, "No. of Z Steps"=w696:u16)
              n486 = Send Notification(notification=w690, notifier=w692) -> ()  [unwired: 1 in, 2 out]
              n487 = Equal To 0?(x=w697) -> (x = 0?=w700:bool)
              n488 = Less?(x=w696, y=u16 2) -> (x < y?=w699:bool)
              n489 = Compound Arithmetic op=OR(w700, w699, w684) -> (w695:bool)
              n490 = case shown="False" w695 {
                tunnel: w703 -> [w706 _]
                tunnel: w693 -> [w708 _]
                frame False {
                  n491 = Obtain Notifier(name (unnamed)="WFDC External Sync", notification data type=T24 {"Cycle Sync"=enum."Pause Requested", "Z Offset"=0.0, "WFDC Status"=enum."Idle"} ("WFDC External Sync"), create if not found? (T)=FALSE) -> (notifier out=w714:refnum<notifier>, error out=w720:errorcluster)  [unwired: 1 in, 1 out]
                  n492 = Get Notifier Status(notifier=w714, error in (no error)=w720) -> (notifier out=w709:refnum<notifier>, current notification=w707:T24, error out=w719:errorcluster)  [unwired: 2 out]
                  n493 = Unbundle By Name(w707) -> ("WFDC Status"=w715:T23)
                  n494 = Unbundle By Name(w719) -> ("status"=w718:bool)
                  n495 = Not Equal?(x=WFDC_Status."DC Active", y=w715) -> (x != y?=w717:bool)
                  n496 = Or(x=w717, y=w718) -> (x .or. y?=w710:bool)
                  n497 = case shown="True" w710 {
                    tunnel: w709 -> [w724 _]
                    tunnel: w708 -> [_ w729]
                    tunnel: w707 -> [w723 _]
                    tunnel: w706 -> [_ w728]
                    tunnel: [u32 350 ("milliseconds to wait") u32 100 ("milliseconds to wait")] -> w705
                    frame False {
                      n498 = Bundle By Name(cluster=w723, "Z Offset"=0.0) -> (w726:T24)
                      n499 = Send Notification(notification=w726, notifier=w724) -> (notifier out=w725:refnum<notifier>)  [unwired: 1 in, 1 out]
                      n500 = Release Notifier(notifier=w725) -> ()  [unwired: 2 in, 3 out]
                    }
                    frame True {
                      n501 = Build Array(w729) -> (w730:dbl[])
                      n502 = call "Stages Messenger.vi"("Stage Notifier Name"=w728, "Actions"=Stage_Actions."MOVE", "Setpoint"=w730, "Axis"=bool[] [TRUE], "Exit While Busy?"=FALSE) -> ()  [unwired: 7 in, 4 out]
                    }
                  }
                  n503 = Wait (ms)(milliseconds to wait=w705) -> ()  [unwired: 1 out]
                }
                frame True {
                }
              }
            }
            frame "External Cycle Sync" {
              n504 = Obtain Notifier(name (unnamed)="WFDC External Sync", notification data type=T24 {"Cycle Sync"=enum."Pause Requested", "Z Offset"=0.0, "WFDC Status"=enum."Idle"} ("WFDC External Sync"), create if not found? (T)=FALSE) -> (notifier out=w752:refnum<notifier>, error out=w755:errorcluster)  [unwired: 1 in, 1 out]
              n505 = Get Notifier Status(notifier=w752, error in (no error)=w755) -> (notifier out=w741:refnum<notifier>, current notification=w740:T24, error out=w754:errorcluster)  [unwired: 2 out]
              n506 = Unbundle By Name(w754) -> ("status"=w748:bool)
              n507 = Unbundle By Name(w740) -> ("WFDC Status"=w739:T23, "Cycle Sync"=w747:T25)
              n508 = Not(x=w748) -> (.not. x?=w743:bool)
              n509 = Equal?(x=WFDC_Status."Error", y=w739) -> (x = y?=w735:bool)
              n510 = Equal?(x=WFDC_Status."DC Active", y=w739) -> (x = y?=w745:bool)
              n511 = Equal?(x=w747, y=WFDC_Cycle_Pause."Pause Requested") -> (x = y?=w744:bool)
              n512 = Compound Arithmetic op=AND(w745, w744, w743) -> (w742:bool)
              n513 = case shown="True" w742 {
                tunnel: w741 -> [_ w765]
                tunnel: w740 -> [_ w767]
                frame False {
                }
                frame True {
                  n514 = Bundle By Name(cluster=w767, "Cycle Sync"=WFDC_Cycle_Pause."Paused") -> (w764:T24)
                  n515 = Send Notification(notification=w764, notifier=w765) -> (notifier out=w763:refnum<notifier>)  [unwired: 1 in, 1 out]
                  n516 = while {
                    tunnel: w763 -> [w778]
                    tunnel: [w769] -> w760
                    tunnel: [w768] -> w762
                    i -> [w774]
                    stop <- w770 stop-if-true
                    n517 = Get Notifier Status(notifier=w778) -> (notifier out=w769:refnum<notifier>, current notification=w768:T24)  [unwired: 1 in, 3 out]
                    n518 = Greater?(x=w774, y=15000) -> (0:w771:bool)
                    n519 = Unbundle By Name(w768) -> ("Cycle Sync"=w777:T25)
                    n520 = Equal?(x=w777, y=WFDC_Cycle_Pause."Resume Requested") -> (x = y?=w772:bool)
                    n521 = Or(x=w772, y=w771) -> (x .or. y?=w770:bool)
                    n522 = Wait (ms)(milliseconds to wait=u32 1) -> ()  [unwired: 1 out]
                  }
                  n523 = Bundle By Name(cluster=w762, "Cycle Sync"=WFDC_Cycle_Pause."Resumed") -> (w759:T24)
                  n524 = Send Notification(notification=w759, notifier=w760) -> (notifier out=w758:refnum<notifier>)  [unwired: 1 in, 1 out]
                  n525 = Release Notifier(notifier=w758) -> ()  [unwired: 2 in, 3 out]
                }
              }
              n526 = Select(t=Orca_Flash_Capture_Actions."Abort" ("y"), s=w735, f=Orca_Flash_Capture_Actions."Setup" ("y")) -> (s? t:f=w736:T12)
            }
            frame "Quit" {
              w788 = FALSE ("Capture?")
              n527 = Get Notifier Status(notifier=w779) -> (notifier out=w783:refnum<notifier>, current notification=w782:T11)  [unwired: 1 in, 3 out]
              n528 = Bundle By Name(cluster=w782, "Running?"=FALSE) -> (w780:T11)
              n529 = Send Notification(notification=w780, notifier=w783) -> ()  [unwired: 1 in, 2 out]
              n530 = Get Notifier Status(notifier=w784) -> (notifier out=w787:refnum<notifier>, current notification=w786:T8)  [unwired: 1 in, 3 out]
              n531 = Bundle By Name(cluster=w786, "Camera Running?"=w788, "Capture?"=w788) -> (w785:T8)
              n532 = Send Notification(notification=w785, notifier=w787) -> ()  [unwired: 1 in, 2 out]
            }
          }
        }
      }
      n533 = local write "Quit"(w239) -> ()
      n534 = Release Notifier(notifier=w199) -> ()  [unwired: 2 in, 3 out]
      n535 = Release Queue(queue=w190) -> ()  [unwired: 2 in, 3 out]
    }
    frame Error {
      n536 = Release Notifier(notifier=w1194) -> (error out=w1193:errorcluster)  [unwired: 2 in, 2 out]
      n537 = for {
        tunnel: w1192 -> [w1199] mode=indexing
        n538 = call "IMAQ Dispose"("Image"=w1199) -> ()  [unwired: 5 in, 1 out]
      }
      n539 = Unbundle By Name(w1193) -> ("source"=w1196:string)
      n540 = Concatenate Strings("4Pi Capture Manager could not start.", "\r", w1196) -> (w1195:string)
      n541 = One Button Dialog(message=w1195) -> ()  [unwired: 1 in, 1 out]
    }
  }
  n542 = control-ref of="This VI"() -> (w109:refnum<vi>)
  n543 = property class="VI"(reference=w109) -> (reference out=w118:refnum<vi>, "Panel"=w110:refnum<vi>)  [unwired: 1 in, 1 out]
  n544 = property class="Pnl"(reference=w110) -> ("Decos[]"=w108:refnum<vi>[], "Panes[]"=w114:refnum<vi>[])  [unwired: 1 in, 2 out]
  n545 = Array Size(array=w108) -> (size(s)=w106:i32)
  n546 = Decrement(x=w106) -> (x-1=w107:i32)
  n547 = Index Array(array=w114, index=0) -> (element=w113:refnum<vi>)
  n548 = Index Array(array=w108, index=w107) -> (element=w116:refnum<vi>)
  n549 = property class="VI"(reference=w118) -> (reference out=w120:refnum<vi>, "Front Panel.PanelBounds"=w121:T32)  [unwired: 1 in, 1 out]
  n550 = property class="Decor"(reference=w116) -> ("Bounds"=w119:T33)  [unwired: 1 in, 2 out]
  n551 = property class="Pane"(reference=w113, "Origin"=T14 {"Horizontal"=0, "Vertical"=0}, "HorizScrollbarVisibility"=w117, "VertScrollbarVisibility"=w117) -> ()  [unwired: 1 in, 2 out]
  n552 = Unbundle By Name(w119) -> ("Width"=w124:u32, "Height"=w127:u32)
  n553 = control-ref of="Quit"() -> (w111:refnum<vi>)
  n554 = To Word Integer(number=w124) -> (16bit integer=w126:i16)
  n555 = To Word Integer(number=w127) -> ()  [unwired: 1 out]
  n556 = property class="Bool (strict)"(reference=w111) -> ("Height"=w129:u32, "Top"=w130:i32)  [unwired: 1 in, 2 out]
  n557 = Unbundle By Name(w121) -> ("Left"=w123:i16, "Top"=w134:i16)
  n558 = To Word Integer(number=w129) -> (16bit integer=w132:i16)
  n559 = To Word Integer(number=w130) -> (16bit integer=w133:i16)
  n560 = Add(x=w123, y=w126) -> (x+y=w125:i16)
  n561 = Compound Arithmetic op=ADD(w134, w132, w133, i16 12 ("y")) -> (w128:i16)
  n562 = Bundle By Name(cluster=w121, "Right"=w125, "Bottom"=w128) -> (w122:T32)
  n563 = property class="VI"(reference=w120, "Front Panel.PanelBounds"=w122) -> ()  [unwired: 1 in, 2 out]
